vi "Main8.vi"() -> ()   [LabVIEW 2017]
uses:
  <vilib>/Analysis/2dsp.llb/Real FFT.vi
  <vilib>/Analysis/NI_AALPro.lvlib
  Atmcd32d.dll
panel:
  in  "index (row)":i32
  out "Angle Integrated Spectrum 2":T1(graph)
  in  "Area Parameteres":T2={"Center angle (deg)"=90.0, "Arc length (deg)"=90.0, "Angle step (deg)"=10.0, "Outer radius "=0.7640449438202247, "Inner radius "=0.0, "Radius"=0.0, "Radial step "=0.5}
  in  "Tab Control":T3(tab)
  out "Current angle":dbl
  in  "Exposure time [ms]":u32=100
  out "Count":i32
  in  "Integration time [s]":dbl=1.0
  out "Ready":bool
  out "Connected":bool
  out "Device":refnum<visa-resource-name>
  in  "Exit":bool
  in  "Take image":bool
  in  "Spectrum":T4(tab)
  out "Fully Integrated Spectrum":dbl(graph)
  out "Angular distribution":dbl[][](graph)
  out "Angle Integrated Spectrum":T5(graph)
  out "Angular distribution 2":dbl[][](graph)
  in  "Energy/Radius":enum32{"Radius", "Energy"}(radio)
  out "Spectrogram up":dbl[][](graph)=[[0.0010313840536425023, 0.0010313840536425023, 0.0010274759814052766, 0.0010401531177745159, 0.00104452387932524, 0.0010522711712232782, 0.001047206375702307, 0.0010453914217880493, 0.0010393489196820073, 0.0010272942106035452, 0.0010408196107141979, 0.0010468510964080136, 0.001062026204249532, 0.001106433361933133, 0.001154520001300267, 0.0011934960677563772, 0.001214033414248973, 0.0012241024150236718, 0.0012391453259184763, 0.0012555680424446059, 0.0012925281054633312, 0.001352528994653044, 0.0014089853532089937, 0.0014660421062312687, 0.0015363130457188075, 0.0015691474623588406, 0.0016108363203256395, 0.0016140062929437132, 0.0015863330654316305, 0.001566139981821102, 0.0015480455247396548, 0.0015630250912641588, 0.0016089194645982896, 0.0016388896140595243, 0.0016752961023638853, 0.001688323009821305, 0.0016919033437948032, 0.0017147706614732288, 0.0017464097973867246, 0.001779717919752482, 0.001837171263614898, 0.00188523587015758, 0.001909243386501412, 0.0019293676175355272, 0.0019505631946586353, 0.0019533283141273984, 0.001977616748982997, 0.0019911972311547808, 0.002017708227177005, 0.002053718124641225, 0.0020883013967221585, 0.002112669700566397, 0.0021315656016372966, 0.0021208218456137463, 0.002105299720787104, 0.002099830072116822, 0.0021012126318512036, 0.0020908214010188896, 0.002095054457416787, 0.002100080695494967, 0.0021084586769929523, 0.0020993728910094368, 0.002104955457905037, 0.0020792872174181134, 0.0020928346503532183, 0.0020942117018814864, 0.002102964241395161, 0.0021093372358679877, 0.002121036665652156, 0.002136567052787968, 0.002154127213876447, 0.002169360157882152, 0.0021869395976920275, 0.0021825908689657556, 0.002171045668952753, 0.0021674267775364637, 0.0021489908116760054, 0.002157660728097984, 0.002145658346977596, 0.002135917084466625, 0.00209696855904108, 0.0020850653256307278, 0.0020535996982097935, 0.002049595232365589, 0.0020524236962046524, 0.0020767176392663643, 0.002111884781195284, 0.002137809153266466, 0.0021668842192343256, 0.00216397037820051, 0.0021656008072099796, 0.0021352698702483386, 0.0021013916485498785, 0.0020823029602650214, 0.0020479290000163844, 0.0020333460243320213, 0.0020002169186649392, 0.0019659586307446764, 0.0019358700548520106, 0.0019274369912928948, 0.0019173046461478957, 0.001900014387158957, 0.0018599917615413628, 0.001814549061108504, 0.0017608991335671654, 0.0017321325271416374, 0.0017011240808280886, 0.0016809695546603515, 0.0016804848325224012, 0.001677022924980334, 0.0016912533754734602, 0.0016999535870290603, 0.0017145172839920274, 0.001701024933118053, 0.0017087557003977521, 0.0017038864461937952, 0.0017154509249281934, 0.0017378638156022909, 0.001773105318313737, 0.0017971238510697952, 0.001824766783448256, 0.0018273914436611356, 0.0018233456662710829, 0.001811169776658133, 0.001808649772361402, 0.0017980740166243004, 0.0017838545825434003, 0.001763256645783561, 0.0017210445082360198, 0.001701132343137258, 0.0016754062664861471, 0.001664623953019805, 0.0016487024832499652, 0.0016273141189128994, 0.0016010950578146683, 0.0015728930425157306, 0.0015352912734848325, 0.0015149109108664593, 0.001483448037548582, 0.0014523514599372237, 0.0014315579818603703, 0.0014274984339550348, 0.0014181675327994876, 0.0014143999198181453, 0.0014053113797315735, 0.0013993515007172275, 0.001408693418285001, 0.0013985390403155494, 0.001397974449188959, 0.0013917694550025816, 0.0013787315311329358, 0.0013626448151797038, 0.0013449083914956062, 0.0013370509354753064, 0.001325880293477993, 0.0013185543793476045, 0.001294420174263172, 0.00127875483607759, 0.0012659041912157889, 0.0012433398248735822, 0.001228894554342046, 0.0012003400138518715, 0.001183988904005212, 0.0011747543964566436, 0.0011585547622780935, 0.0011605046672421217, 0.0011473565792502146, 0.0011370039058606926, 0.0011340652778993677, 0.0011226770617605876, 0.0011216442731143861, 0.0011107600578349525, 0.0011026409620242816, 0.0010866919512238764, 0.0010731362559796018, 0.001051089661012024, 0.0010301832647098524, 0.001009888279286232, 0.0009965887156262153, 0.0009909235256389188, 0.0009767536654130364, 0.0009747817276245561, 0.0009568910741692924, 0.000949947980363763, 0.000956703795161448, 0.0009593917997446279, 0.0009746082191319944, 0.0009815127554947322, 0.0009862085012061277, 0.0009848589907084247, 0.0009587748806599638, 0.0009397330121270677, 0.0009244532483694009, 0.0009160174307072283, 0.0009138141482619988, 0.0009141501488348964, 0.0009184162544694721, 0.0009130457535092251, 0.000912208506180038, 0.0009004897976744733, 0.0008954966088329721, 0.000888658170943591, 0.000878327530378521, 0.0008779392018475493, 0.0008724833236925496, 0.0008753007711193868, 0.0008733894235981503, 0.0008842763929806406, 0.0008803270091975667, 0.0008834474079606231, 0.0008812331091031674, 0.0008784927765619131, 0.0008838109495640858, 0.0008909550928927427, 0.000899184352825675, 0.0009081654828930417, 0.000914194214483801, 0.0009259542345352136, 0.0009387635678511666, 0.0009425339349355657, 0.0009425063939050002, 0.0009326494590656548, 0.0009267529244216092, 0.0009192645182108854, 0.0009126023429171226, 0.0009054058716303917, 0.0008956756255316468, 0.0008975015958581308, 0.0008902445343041561, 0.0008840973762819658, 0.0008824283898297043, 0.0008799772381093866, 0.000884678492026895, 0.0008933897199947213, 0.0008983829088362226, 0.000893860671617389, 0.0008973749071175302, 0.0009013435696219998, 0.0009055848883290665, 0.0009138995254567515, 0.0009202174378684471, 0.000930589389979365, 0.000922150818214136, 0.0009280666315795773, 0.0009267253833910438, 0.0009243623629685353, 0.0009317653919845064, 0.0009418922289233926, 0.0009494384712983037, 0.0009643051195974898, 0.0009718458537662879, 0.0009862966325039368, 0.0009917001827008621, 0.0009979795376697665, 0.001014038712592433, 0.0010172830459930335, 0.0010330585483008768, 0.0010469640146333317, 0.001060098332109956, 0.0010826544361429932, 0.0011030761103072145, 0.0011350760337211167, 0.0011531154087414334, 0.0011576624328877758, 0.0011768364983673857, 0.0011841624124977737, 0.0011999406689086737, 0.0012165093528967996, 0.0012281895039595726, 0.0012561601746017613, 0.0012707651831105765, 0.001307240523991351, 0.001333627585376031, 0.0013666217399933432, 0.0014024911782016796, 0.0014332324765187446, 0.0014678102403935655, 0.0014988241949132272, 0.0015329365153714935, 0.0015343879276822883, 0.0015720971067323913, 0.0016118636007657278, 0.001651087536496926, 0.0016970920739533186, 0.001745473402347502, 0.0017665615694514051, 0.0018051024876245825, 0.0018256783915599696, 0.0018815618966801597, 0.0018972630382054765, 0.0019475088943689358, 0.001967589059754146, 0.0019944801219981727, 0.0020293085092511383, 0.0020797967264835726, 0.002127649267090901, 0.002177592171918141, 0.002209096356781867, 0.0022576126362258207, 0.0022860239633570555, 0.002367479315357191, 0.00239798651491445, 0.002459918030346795, 0.002492961758819125, 0.0025305745442622493, 0.0025619850896220525, 0.0025918974029190997, 0.0026126908809959533, 0.0026649499864937407, 0.002671884817990101, 0.0027487573425041584, 0.0027664331759210126, 0.0028080311484869457, 0.002835572179052315, 0.002897776350687257, 0.0029281981730497637, 0.0029626547563900967, 0.002993387792397992, 0.0030170785868903222, 0.0030149964849795806, 0.0030319039236436605, 0.0030360240618162396, 0.0030334957952103388, 0.0030378693108641195, 0.003026379192912247, 0.0030242502712495446, 0.0030348563221202682, 0.0030418489897808152, 0.0030719182869520852, 0.0030982750532031434, 0.0030908086798168716, 0.0031010319103627363, 0.0031036813575031253, 0.0030762670156783568, 0.003066933360419753, 0.003042223547796504, 0.0030263378813663996, 0.003004663090311454, 0.0029920548065186284, 0.0029706664421815625, 0.0029578268137319874, 0.0029413352446294445, 0.0029132489016588815, 0.0028961762168114094, 0.002857943758180564, 0.00283680050901553, 0.0028030104186148787, 0.0027938640423641197, 0.0027516161014768444, 0.002719478472910115, 0.0026733913123620267, 0.002627637398283779, 0.0025728335015617514, 0.0025436510255746865, 0.002504355483164018, 0.0024615594757684913, 0.002436053727361903, 0.0024182842544411267, 0.0024007185851465346, 0.0023905779776923655, 0.0023550968680150007, 0.002333292634116398, 0.002292746728918062, 0.0022553735504408563, 0.0022384468330553806, 0.002203128215458351, 0.00217902430550754, 0.002143711196116624, 0.0021122262899742946, 0.0020506142504965077, 0.00203825383597877, 0.0020262487007553258, 0.0020074629638066875, 0.0019932738248594093, 0.0019544327094530695, 0.0019488088310116213, 0.0019049882972790627, 0.0018915620448784454, 0.0018528393559035367, 0.001821197465886984, 0.0017890212798774634, 0.0017354539754278208, 0.0016897689139259869, 0.001663423164087155, 0.0016456371665480398, 0.0016412085688331283, 0.001628644350689207, 0.0016130809143167168, 0.0016073331012377244, 0.001603339651805746, 0.0015941712427305346, 0.001588935692820058, 0.0015824029603699523, 0.00157714813173808, 0.0015643332902160138, 0.0015630746651191763, 0.0015527274999357675, 0.0015555421932595482, 0.0015637163711313498, 0.0015732180266764021, 0.001592557338339404, 0.001584653062567143, 0.0015960522951181493, 0.0016165015103129358, 0.0016268707083207973, 0.0016398039762742945, 0.001641899848700319, 0.0016484215647381982, 0.0016487190078683044, 0.0016555629539637985, 0.0016557612493838694, 0.0016741145921526312, 0.0017004658501975761, 0.0017330110860166727, 0.0017605190673453631, 0.0017664348807108045, 0.0017779084740443371, 0.001790398331405732, 0.0018131775177863488, 0.0018366452299310996, 0.0018605453362557267, 0.0018882543671075445, 0.0018984252696953353, 0.001914192509694009, 0.0019416316384462862, 0.0019781785860065308, 0.0020108477564631713, 0.0020298097560074277, 0.0020661143424986973, 0.002068810609391047, 0.002110609631480107, 0.002115869968318093, 0.0021256800834054774, 0.0021556667574850513, 0.002178443189762611, 0.0021840174943490416, 0.002213334921385877, 0.002212183706308245, 0.00223874152208243, 0.0022391546375409104, 0.002258397555596934, 0.0022739802706908193, 0.0023094503639559585, 0.002319709397841558, 0.002351866305129683, 0.002368812301236555, 0.0023749456887434623, 0.002389630566240917, 0.0023986777947816403, 0.00241149814450982, 0.0024190003212358263, 0.0024229882624616918, 0.002422095933071374, 0.002423731870286957, 0.0024201625527256847, 0.0024417767535133868, 0.0024415812121963724, 0.002455808908586442, 0.002457513698378438, 0.0024465385976981386, 0.0024522313287160006, 0.0024169705472831585, 0.0024148361174143426, 0.0023995701241719585, 0.0023793853028705996, 0.0023548297200185167, 0.002332361747283289, 0.0023205108418310103, 0.0022940521737668603, 0.0022523164960481005, 0.0022274744864781374, 0.0022039158889325208, 0.0021684926154193433, 0.0021411526343771015, 0.002118635087786856, 0.002083801192327777, 0.002047124801923875, 0.0020278653592495127, 0.0019697703093749233, 0.0019519264756716211, 0.0019212622922401392, 0.0018812286502103187, 0.0018427428140982722, 0.001812265909674635, 0.00175640994558501, 0.0017214080498394828, 0.0016736711815605288, 0.0016349457384825634, 0.0015946835058990505, 0.0015675610989982752, 0.0015259052902681545, 0.0014996366553149056, 0.001476708747369236, 0.001439175830914751, 0.0014011692087345419, 0.0013630882257718063, 0.0013162216540587178, 0.0012905451512626243, 0.0012539458757443056, 0.0012235736272368167, 0.0012001196856073486, 0.001185272316029558, 0.0011544346241055146, 0.0011379100057662933, 0.0010844501113358553, 0.0010647610285846733, 0.0010130802847287583, 0.0009929670701068693, 0.0009656849252288149, 0.0009476042386626501, 0.0009280005331062204, 0.0009123489654359212, 0.0008921173243826012, 0.0008740696870531149, 0.000861342976828858, 0.0008399518583887359, 0.0008269304591374295, 0.000805963472568014, 0.0007840931401960546, 0.0007730684656607372, 0.0007618757908389714, 0.000755502796366145, 0.0007484440302322409, 0.0007361304354664644, 0.0007236515945172958, 0.0007035631668229157, 0.0006909796699575985, 0.0006775396470416985, 0.0006603843391025302, 0.0006506954045496334, 0.0006404831904159946, 0.0006315406177914192, 0.000626814576946402, 0.0006201799426832045, 0.0006156053775062967, 0.0006078663479174281, 0.0005998298751984535, 0.0005900335306263518, 0.0005812644664943382, 0.0005748804556092857, 0.0005698349388097101, 0.000566761359798615, 0.0005616442363195694, 0.0005622749259195163, 0.0005532993040582626, 0.0005422911541412846, 0.0005348495676825219, 0.0005325361211150309, 0.0005320376284617976, 0.0005307018884793774, 0.0005264054877111798, 0.0005264054877111798, 0.0005228637111804734, 0.0005181238998201733, 0.0005176309153730532, 0.0005136154331166225, 0.0005124091359778592, 0.0005101562796776121, 0.0005055431570579128, 0.0004995529829099451, 0.0004920150028442035, 0.0004884759804165536, 0.00048560345092858563, 0.000481450263519328, 0.000479029406932632, 0.00047415189041950524, 0.00047243608421528277, 0.0004715299843096821, 0.00047353772543789753, 0.00047000971942247376, 0.0004698554896513077, 0.0004721276246729506, 0.0004682388311571205, 0.0004696351614067847, 0.0004644106279085342, 0.00046173088563452376, 0.0004594807834373332, 0.0004550053659704607, 0.0004509155229315034, 0.00044808430498938354, 0.0004430277717775818, 0.0004410696045043841, 0.00043787759906185783, 0.00043347929648056836, 0.0004299017166101269, 0.00042542354504019795, 0.00042215993291820175, 0.00041868425486085215, 0.000416883071461877, 0.0004110388647759057, 0.0004118981449295452, 0.00040788541677617095, 0.00040867033614728403, 0.00040761000647051725, 0.0004041866563712419, 0.00040178507850594175, 0.00039903372955246133, 0.0003977007436730975, 0.0003977310388067194, 0.00039884645054461687, 0.00039690480788975835, 0.000394671230310907, 0.0003933712936682215, 0.00039117076532604856, 0.0003899947633209073, 0.00038895095826247983, 0.00038990112381698505, 0.00038822662915861066, 0.0003852577060636639, 0.00038354740806555447, 0.0003831673418437523, 0.00038108523993301045, 0.00038199133983861106, 0.0003807712721845652, 0.0003789921216100424, 0.0003772350038599718, 0.00037759028315426514, 0.0003756155912627282, 0.0003736216206497954, 0.000373136898511845, 0.0003710079768491419, 0.0003707132878220925, 0.0003699917128212798, 0.00036924259678990177, 0.0003697686304737003, 0.000369484957858877, 0.0003692976788510325, 0.00037006056539769325, 0.00036974108944313496, 0.00036845492331573224, 0.0003671825277036122, 0.0003674441674939832, 0.00036729820003198675, 0.00036671708428705744, 0.0003670723635813507, 0.0003662516408705027, 0.0003653593114801848, 0.0003654336722627113, 0.00036621859163382426, 0.0003649076385789127, 0.0003645000313265452, 0.00036404009611610357, 0.00036481399907499045, 0.00036354435756592694, 0.0003624454704463687, 0.00036318632416857717, 0.000362616224835874, 0.00036201858447260554, 0.0003629026515537539, 0.00036316429134412485, 0.0003618092726403087, 0.00036178173160974337, 0.0003609059268377646, 0.0003606580575626763, 0.00035972441662651027, 0.00035978776099681063, 0.0003598290725426587, 0.0003593278257863689, 0.00035902487445014993, 0.0003587962838964574, 0.00035836939792269413, 0.00035583837721373673, 0.0003554059830338604, 0.0003547532606094612, 0.0003549102444836838, 0.00035429057129596295, 0.0003543126041204152, 0.0003549185067928534, 0.0003548248672889311, 0.00035513057272820676, 0.0003544998831282598, 0.00035434014515098067, 0.000354516407746599, 0.00035333489753534467, 0.0003535855209134895, 0.0003530154215807864, 0.0003527152243476239, 0.0003532798154742139, 0.00035263260125592777, 0.0003519964034498677, 0.000351608074918896, 0.00035093882787615757, 0.000349443349916458, 0.00034942957940117537, 0.0003491624314046913, 0.00034956453045094566, 0.00034901095573658175, 0.00034910184113744744, 0.0003489310867479422, 0.0003488181685226241, 0.0003479836752964935, 0.0003476917403725006, 0.00034843259409470895, 0.0003489586277785075, 0.0003480910853156984, 0.0003474548875096384, 0.0003469619030625183, 0.00034665344352018617, 0.0003463918037298151, 0.00034654052529486815, 0.00034605304905386115, 0.0003454196053508576, 0.00034516347376659963, 0.00034559862204953256, 0.0003448357355028718, 0.0003449403914190202, 0.00034430419361296017, 0.00034424635744877293, 0.000344852260121211, 0.0003448384896059283, 0.0003451028834993559, 0.0003437423565894266, 0.0003425580922751158, 0.00034259664971790727, 0.0003416354677511759, 0.00034174838597649394, 0.00034173461546121124, 0.0003417869434192854, 0.0003409965158420593, 0.00034094143378092864, 0.0003408477942770064, 0.0003402501539137379, 0.0003404980231888262, 0.0003398783500011054, 0.00033904936498108774, 0.00033842969179336696, 0.00033828372433137053, 0.0003380661501899041, 0.00033740791955939176, 0.000338358085113897, 0.0003377081167925543, 0.00033727847671573453, 0.000337388640837996, 0.00033701959102842003, 0.00033749605085720095, 0.00033774116602923275, 0.0003364384752834908, 0.000335931720321088, 0.0003357031297673954, 0.00033592070390886183, 0.0003353395881639325, 0.00033492922680850853, 0.00033513303043469225, 0.00033468961984258985, 0.0003348713906443213, 0.00033494024322073466, 0.0003348108003770775, 0.00033487689885043436, 0.00033441145543387964, 0.0003341993894985263, 0.0003345464064836499, 0.00033424896335354395, 0.00033390194636842026, 0.00033334837165405635, 0.00033337040447850867, 0.0003331583385431553, 0.0003329132233711235, 0.0003332326993256818, 0.0003335301424557878, 0.0003335026014252224, 0.00033401761869679484, 0.0003333428634479433, 0.00033282509207331433, 0.00033313630571870306, 0.0003330839777606288, 0.00033270666564188324, 0.00033214758272140626, 0.00033204843501137094, 0.00033124974512497527, 0.0003311781384455053, 0.00033189695934326144, 0.0003313213518044452, 0.0003320980088663886, 0.0003318336149729611, 0.00033207873014499283, 0.0003325304030462649, 0.0003314094831022544, 0.00033175650008737803]]
  out "Range scan":dbl[][](graph)
  out "Spectrogram down":dbl[][](graph)=[[0.0010313840536425023, 0.0010313840536425023, 0.0010274759814052766, 0.0010401531177745159, 0.00104452387932524, 0.0010522711712232782, 0.001047206375702307, 0.0010453914217880493, 0.0010393489196820073, 0.0010272942106035452, 0.0010408196107141979, 0.0010468510964080136, 0.001062026204249532, 0.001106433361933133, 0.001154520001300267, 0.0011934960677563772, 0.001214033414248973, 0.0012241024150236718, 0.0012391453259184763, 0.0012555680424446059, 0.0012925281054633312, 0.001352528994653044, 0.0014089853532089937, 0.0014660421062312687, 0.0015363130457188075, 0.0015691474623588406, 0.0016108363203256395, 0.0016140062929437132, 0.0015863330654316305, 0.001566139981821102, 0.0015480455247396548, 0.0015630250912641588, 0.0016089194645982896, 0.0016388896140595243, 0.0016752961023638853, 0.001688323009821305, 0.0016919033437948032, 0.0017147706614732288, 0.0017464097973867246, 0.001779717919752482, 0.001837171263614898, 0.00188523587015758, 0.001909243386501412, 0.0019293676175355272, 0.0019505631946586353, 0.0019533283141273984, 0.001977616748982997, 0.0019911972311547808, 0.002017708227177005, 0.002053718124641225, 0.0020883013967221585, 0.002112669700566397, 0.0021315656016372966, 0.0021208218456137463, 0.002105299720787104, 0.002099830072116822, 0.0021012126318512036, 0.0020908214010188896, 0.002095054457416787, 0.002100080695494967, 0.0021084586769929523, 0.0020993728910094368, 0.002104955457905037, 0.0020792872174181134, 0.0020928346503532183, 0.0020942117018814864, 0.002102964241395161, 0.0021093372358679877, 0.002121036665652156, 0.002136567052787968, 0.002154127213876447, 0.002169360157882152, 0.0021869395976920275, 0.0021825908689657556, 0.002171045668952753, 0.0021674267775364637, 0.0021489908116760054, 0.002157660728097984, 0.002145658346977596, 0.002135917084466625, 0.00209696855904108, 0.0020850653256307278, 0.0020535996982097935, 0.002049595232365589, 0.0020524236962046524, 0.0020767176392663643, 0.002111884781195284, 0.002137809153266466, 0.0021668842192343256, 0.00216397037820051, 0.0021656008072099796, 0.0021352698702483386, 0.0021013916485498785, 0.0020823029602650214, 0.0020479290000163844, 0.0020333460243320213, 0.0020002169186649392, 0.0019659586307446764, 0.0019358700548520106, 0.0019274369912928948, 0.0019173046461478957, 0.001900014387158957, 0.0018599917615413628, 0.001814549061108504, 0.0017608991335671654, 0.0017321325271416374, 0.0017011240808280886, 0.0016809695546603515, 0.0016804848325224012, 0.001677022924980334, 0.0016912533754734602, 0.0016999535870290603, 0.0017145172839920274, 0.001701024933118053, 0.0017087557003977521, 0.0017038864461937952, 0.0017154509249281934, 0.0017378638156022909, 0.001773105318313737, 0.0017971238510697952, 0.001824766783448256, 0.0018273914436611356, 0.0018233456662710829, 0.001811169776658133, 0.001808649772361402, 0.0017980740166243004, 0.0017838545825434003, 0.001763256645783561, 0.0017210445082360198, 0.001701132343137258, 0.0016754062664861471, 0.001664623953019805, 0.0016487024832499652, 0.0016273141189128994, 0.0016010950578146683, 0.0015728930425157306, 0.0015352912734848325, 0.0015149109108664593, 0.001483448037548582, 0.0014523514599372237, 0.0014315579818603703, 0.0014274984339550348, 0.0014181675327994876, 0.0014143999198181453, 0.0014053113797315735, 0.0013993515007172275, 0.001408693418285001, 0.0013985390403155494, 0.001397974449188959, 0.0013917694550025816, 0.0013787315311329358, 0.0013626448151797038, 0.0013449083914956062, 0.0013370509354753064, 0.001325880293477993, 0.0013185543793476045, 0.001294420174263172, 0.00127875483607759, 0.0012659041912157889, 0.0012433398248735822, 0.001228894554342046, 0.0012003400138518715, 0.001183988904005212, 0.0011747543964566436, 0.0011585547622780935, 0.0011605046672421217, 0.0011473565792502146, 0.0011370039058606926, 0.0011340652778993677, 0.0011226770617605876, 0.0011216442731143861, 0.0011107600578349525, 0.0011026409620242816, 0.0010866919512238764, 0.0010731362559796018, 0.001051089661012024, 0.0010301832647098524, 0.001009888279286232, 0.0009965887156262153, 0.0009909235256389188, 0.0009767536654130364, 0.0009747817276245561, 0.0009568910741692924, 0.000949947980363763, 0.000956703795161448, 0.0009593917997446279, 0.0009746082191319944, 0.0009815127554947322, 0.0009862085012061277, 0.0009848589907084247, 0.0009587748806599638, 0.0009397330121270677, 0.0009244532483694009, 0.0009160174307072283, 0.0009138141482619988, 0.0009141501488348964, 0.0009184162544694721, 0.0009130457535092251, 0.000912208506180038, 0.0009004897976744733, 0.0008954966088329721, 0.000888658170943591, 0.000878327530378521, 0.0008779392018475493, 0.0008724833236925496, 0.0008753007711193868, 0.0008733894235981503, 0.0008842763929806406, 0.0008803270091975667, 0.0008834474079606231, 0.0008812331091031674, 0.0008784927765619131, 0.0008838109495640858, 0.0008909550928927427, 0.000899184352825675, 0.0009081654828930417, 0.000914194214483801, 0.0009259542345352136, 0.0009387635678511666, 0.0009425339349355657, 0.0009425063939050002, 0.0009326494590656548, 0.0009267529244216092, 0.0009192645182108854, 0.0009126023429171226, 0.0009054058716303917, 0.0008956756255316468, 0.0008975015958581308, 0.0008902445343041561, 0.0008840973762819658, 0.0008824283898297043, 0.0008799772381093866, 0.000884678492026895, 0.0008933897199947213, 0.0008983829088362226, 0.000893860671617389, 0.0008973749071175302, 0.0009013435696219998, 0.0009055848883290665, 0.0009138995254567515, 0.0009202174378684471, 0.000930589389979365, 0.000922150818214136, 0.0009280666315795773, 0.0009267253833910438, 0.0009243623629685353, 0.0009317653919845064, 0.0009418922289233926, 0.0009494384712983037, 0.0009643051195974898, 0.0009718458537662879, 0.0009862966325039368, 0.0009917001827008621, 0.0009979795376697665, 0.001014038712592433, 0.0010172830459930335, 0.0010330585483008768, 0.0010469640146333317, 0.001060098332109956, 0.0010826544361429932, 0.0011030761103072145, 0.0011350760337211167, 0.0011531154087414334, 0.0011576624328877758, 0.0011768364983673857, 0.0011841624124977737, 0.0011999406689086737, 0.0012165093528967996, 0.0012281895039595726, 0.0012561601746017613, 0.0012707651831105765, 0.001307240523991351, 0.001333627585376031, 0.0013666217399933432, 0.0014024911782016796, 0.0014332324765187446, 0.0014678102403935655, 0.0014988241949132272, 0.0015329365153714935, 0.0015343879276822883, 0.0015720971067323913, 0.0016118636007657278, 0.001651087536496926, 0.0016970920739533186, 0.001745473402347502, 0.0017665615694514051, 0.0018051024876245825, 0.0018256783915599696, 0.0018815618966801597, 0.0018972630382054765, 0.0019475088943689358, 0.001967589059754146, 0.0019944801219981727, 0.0020293085092511383, 0.0020797967264835726, 0.002127649267090901, 0.002177592171918141, 0.002209096356781867, 0.0022576126362258207, 0.0022860239633570555, 0.002367479315357191, 0.00239798651491445, 0.002459918030346795, 0.002492961758819125, 0.0025305745442622493, 0.0025619850896220525, 0.0025918974029190997, 0.0026126908809959533, 0.0026649499864937407, 0.002671884817990101, 0.0027487573425041584, 0.0027664331759210126, 0.0028080311484869457, 0.002835572179052315, 0.002897776350687257, 0.0029281981730497637, 0.0029626547563900967, 0.002993387792397992, 0.0030170785868903222, 0.0030149964849795806, 0.0030319039236436605, 0.0030360240618162396, 0.0030334957952103388, 0.0030378693108641195, 0.003026379192912247, 0.0030242502712495446, 0.0030348563221202682, 0.0030418489897808152, 0.0030719182869520852, 0.0030982750532031434, 0.0030908086798168716, 0.0031010319103627363, 0.0031036813575031253, 0.0030762670156783568, 0.003066933360419753, 0.003042223547796504, 0.0030263378813663996, 0.003004663090311454, 0.0029920548065186284, 0.0029706664421815625, 0.0029578268137319874, 0.0029413352446294445, 0.0029132489016588815, 0.0028961762168114094, 0.002857943758180564, 0.00283680050901553, 0.0028030104186148787, 0.0027938640423641197, 0.0027516161014768444, 0.002719478472910115, 0.0026733913123620267, 0.002627637398283779, 0.0025728335015617514, 0.0025436510255746865, 0.002504355483164018, 0.0024615594757684913, 0.002436053727361903, 0.0024182842544411267, 0.0024007185851465346, 0.0023905779776923655, 0.0023550968680150007, 0.002333292634116398, 0.002292746728918062, 0.0022553735504408563, 0.0022384468330553806, 0.002203128215458351, 0.00217902430550754, 0.002143711196116624, 0.0021122262899742946, 0.0020506142504965077, 0.00203825383597877, 0.0020262487007553258, 0.0020074629638066875, 0.0019932738248594093, 0.0019544327094530695, 0.0019488088310116213, 0.0019049882972790627, 0.0018915620448784454, 0.0018528393559035367, 0.001821197465886984, 0.0017890212798774634, 0.0017354539754278208, 0.0016897689139259869, 0.001663423164087155, 0.0016456371665480398, 0.0016412085688331283, 0.001628644350689207, 0.0016130809143167168, 0.0016073331012377244, 0.001603339651805746, 0.0015941712427305346, 0.001588935692820058, 0.0015824029603699523, 0.00157714813173808, 0.0015643332902160138, 0.0015630746651191763, 0.0015527274999357675, 0.0015555421932595482, 0.0015637163711313498, 0.0015732180266764021, 0.001592557338339404, 0.001584653062567143, 0.0015960522951181493, 0.0016165015103129358, 0.0016268707083207973, 0.0016398039762742945, 0.001641899848700319, 0.0016484215647381982, 0.0016487190078683044, 0.0016555629539637985, 0.0016557612493838694, 0.0016741145921526312, 0.0017004658501975761, 0.0017330110860166727, 0.0017605190673453631, 0.0017664348807108045, 0.0017779084740443371, 0.001790398331405732, 0.0018131775177863488, 0.0018366452299310996, 0.0018605453362557267, 0.0018882543671075445, 0.0018984252696953353, 0.001914192509694009, 0.0019416316384462862, 0.0019781785860065308, 0.0020108477564631713, 0.0020298097560074277, 0.0020661143424986973, 0.002068810609391047, 0.002110609631480107, 0.002115869968318093, 0.0021256800834054774, 0.0021556667574850513, 0.002178443189762611, 0.0021840174943490416, 0.002213334921385877, 0.002212183706308245, 0.00223874152208243, 0.0022391546375409104, 0.002258397555596934, 0.0022739802706908193, 0.0023094503639559585, 0.002319709397841558, 0.002351866305129683, 0.002368812301236555, 0.0023749456887434623, 0.002389630566240917, 0.0023986777947816403, 0.00241149814450982, 0.0024190003212358263, 0.0024229882624616918, 0.002422095933071374, 0.002423731870286957, 0.0024201625527256847, 0.0024417767535133868, 0.0024415812121963724, 0.002455808908586442, 0.002457513698378438, 0.0024465385976981386, 0.0024522313287160006, 0.0024169705472831585, 0.0024148361174143426, 0.0023995701241719585, 0.0023793853028705996, 0.0023548297200185167, 0.002332361747283289, 0.0023205108418310103, 0.0022940521737668603, 0.0022523164960481005, 0.0022274744864781374, 0.0022039158889325208, 0.0021684926154193433, 0.0021411526343771015, 0.002118635087786856, 0.002083801192327777, 0.002047124801923875, 0.0020278653592495127, 0.0019697703093749233, 0.0019519264756716211, 0.0019212622922401392, 0.0018812286502103187, 0.0018427428140982722, 0.001812265909674635, 0.00175640994558501, 0.0017214080498394828, 0.0016736711815605288, 0.0016349457384825634, 0.0015946835058990505, 0.0015675610989982752, 0.0015259052902681545, 0.0014996366553149056, 0.001476708747369236, 0.001439175830914751, 0.0014011692087345419, 0.0013630882257718063, 0.0013162216540587178, 0.0012905451512626243, 0.0012539458757443056, 0.0012235736272368167, 0.0012001196856073486, 0.001185272316029558, 0.0011544346241055146, 0.0011379100057662933, 0.0010844501113358553, 0.0010647610285846733, 0.0010130802847287583, 0.0009929670701068693, 0.0009656849252288149, 0.0009476042386626501, 0.0009280005331062204, 0.0009123489654359212, 0.0008921173243826012, 0.0008740696870531149, 0.000861342976828858, 0.0008399518583887359, 0.0008269304591374295, 0.000805963472568014, 0.0007840931401960546, 0.0007730684656607372, 0.0007618757908389714, 0.000755502796366145, 0.0007484440302322409, 0.0007361304354664644, 0.0007236515945172958, 0.0007035631668229157, 0.0006909796699575985, 0.0006775396470416985, 0.0006603843391025302, 0.0006506954045496334, 0.0006404831904159946, 0.0006315406177914192, 0.000626814576946402, 0.0006201799426832045, 0.0006156053775062967, 0.0006078663479174281, 0.0005998298751984535, 0.0005900335306263518, 0.0005812644664943382, 0.0005748804556092857, 0.0005698349388097101, 0.000566761359798615, 0.0005616442363195694, 0.0005622749259195163, 0.0005532993040582626, 0.0005422911541412846, 0.0005348495676825219, 0.0005325361211150309, 0.0005320376284617976, 0.0005307018884793774, 0.0005264054877111798, 0.0005264054877111798, 0.0005228637111804734, 0.0005181238998201733, 0.0005176309153730532, 0.0005136154331166225, 0.0005124091359778592, 0.0005101562796776121, 0.0005055431570579128, 0.0004995529829099451, 0.0004920150028442035, 0.0004884759804165536, 0.00048560345092858563, 0.000481450263519328, 0.000479029406932632, 0.00047415189041950524, 0.00047243608421528277, 0.0004715299843096821, 0.00047353772543789753, 0.00047000971942247376, 0.0004698554896513077, 0.0004721276246729506, 0.0004682388311571205, 0.0004696351614067847, 0.0004644106279085342, 0.00046173088563452376, 0.0004594807834373332, 0.0004550053659704607, 0.0004509155229315034, 0.00044808430498938354, 0.0004430277717775818, 0.0004410696045043841, 0.00043787759906185783, 0.00043347929648056836, 0.0004299017166101269, 0.00042542354504019795, 0.00042215993291820175, 0.00041868425486085215, 0.000416883071461877, 0.0004110388647759057, 0.0004118981449295452, 0.00040788541677617095, 0.00040867033614728403, 0.00040761000647051725, 0.0004041866563712419, 0.00040178507850594175, 0.00039903372955246133, 0.0003977007436730975, 0.0003977310388067194, 0.00039884645054461687, 0.00039690480788975835, 0.000394671230310907, 0.0003933712936682215, 0.00039117076532604856, 0.0003899947633209073, 0.00038895095826247983, 0.00038990112381698505, 0.00038822662915861066, 0.0003852577060636639, 0.00038354740806555447, 0.0003831673418437523, 0.00038108523993301045, 0.00038199133983861106, 0.0003807712721845652, 0.0003789921216100424, 0.0003772350038599718, 0.00037759028315426514, 0.0003756155912627282, 0.0003736216206497954, 0.000373136898511845, 0.0003710079768491419, 0.0003707132878220925, 0.0003699917128212798, 0.00036924259678990177, 0.0003697686304737003, 0.000369484957858877, 0.0003692976788510325, 0.00037006056539769325, 0.00036974108944313496, 0.00036845492331573224, 0.0003671825277036122, 0.0003674441674939832, 0.00036729820003198675, 0.00036671708428705744, 0.0003670723635813507, 0.0003662516408705027, 0.0003653593114801848, 0.0003654336722627113, 0.00036621859163382426, 0.0003649076385789127, 0.0003645000313265452, 0.00036404009611610357, 0.00036481399907499045, 0.00036354435756592694, 0.0003624454704463687, 0.00036318632416857717, 0.000362616224835874, 0.00036201858447260554, 0.0003629026515537539, 0.00036316429134412485, 0.0003618092726403087, 0.00036178173160974337, 0.0003609059268377646, 0.0003606580575626763, 0.00035972441662651027, 0.00035978776099681063, 0.0003598290725426587, 0.0003593278257863689, 0.00035902487445014993, 0.0003587962838964574, 0.00035836939792269413, 0.00035583837721373673, 0.0003554059830338604, 0.0003547532606094612, 0.0003549102444836838, 0.00035429057129596295, 0.0003543126041204152, 0.0003549185067928534, 0.0003548248672889311, 0.00035513057272820676, 0.0003544998831282598, 0.00035434014515098067, 0.000354516407746599, 0.00035333489753534467, 0.0003535855209134895, 0.0003530154215807864, 0.0003527152243476239, 0.0003532798154742139, 0.00035263260125592777, 0.0003519964034498677, 0.000351608074918896, 0.00035093882787615757, 0.000349443349916458, 0.00034942957940117537, 0.0003491624314046913, 0.00034956453045094566, 0.00034901095573658175, 0.00034910184113744744, 0.0003489310867479422, 0.0003488181685226241, 0.0003479836752964935, 0.0003476917403725006, 0.00034843259409470895, 0.0003489586277785075, 0.0003480910853156984, 0.0003474548875096384, 0.0003469619030625183, 0.00034665344352018617, 0.0003463918037298151, 0.00034654052529486815, 0.00034605304905386115, 0.0003454196053508576, 0.00034516347376659963, 0.00034559862204953256, 0.0003448357355028718, 0.0003449403914190202, 0.00034430419361296017, 0.00034424635744877293, 0.000344852260121211, 0.0003448384896059283, 0.0003451028834993559, 0.0003437423565894266, 0.0003425580922751158, 0.00034259664971790727, 0.0003416354677511759, 0.00034174838597649394, 0.00034173461546121124, 0.0003417869434192854, 0.0003409965158420593, 0.00034094143378092864, 0.0003408477942770064, 0.0003402501539137379, 0.0003404980231888262, 0.0003398783500011054, 0.00033904936498108774, 0.00033842969179336696, 0.00033828372433137053, 0.0003380661501899041, 0.00033740791955939176, 0.000338358085113897, 0.0003377081167925543, 0.00033727847671573453, 0.000337388640837996, 0.00033701959102842003, 0.00033749605085720095, 0.00033774116602923275, 0.0003364384752834908, 0.000335931720321088, 0.0003357031297673954, 0.00033592070390886183, 0.0003353395881639325, 0.00033492922680850853, 0.00033513303043469225, 0.00033468961984258985, 0.0003348713906443213, 0.00033494024322073466, 0.0003348108003770775, 0.00033487689885043436, 0.00033441145543387964, 0.0003341993894985263, 0.0003345464064836499, 0.00033424896335354395, 0.00033390194636842026, 0.00033334837165405635, 0.00033337040447850867, 0.0003331583385431553, 0.0003329132233711235, 0.0003332326993256818, 0.0003335301424557878, 0.0003335026014252224, 0.00033401761869679484, 0.0003333428634479433, 0.00033282509207331433, 0.00033313630571870306, 0.0003330839777606288, 0.00033270666564188324, 0.00033214758272140626, 0.00033204843501137094, 0.00033124974512497527, 0.0003311781384455053, 0.00033189695934326144, 0.0003313213518044452, 0.0003320980088663886, 0.0003318336149729611, 0.00033207873014499283, 0.0003325304030462649, 0.0003314094831022544, 0.00033175650008737803]]
  out "FFT":dbl[](graph)
  out "Asymetry spectrogarm":dbl[][](graph)=[[0.0010313840536425023, 0.0010313840536425023, 0.0010274759814052766, 0.0010401531177745159, 0.00104452387932524, 0.0010522711712232782, 0.001047206375702307, 0.0010453914217880493, 0.0010393489196820073, 0.0010272942106035452, 0.0010408196107141979, 0.0010468510964080136, 0.001062026204249532, 0.001106433361933133, 0.001154520001300267, 0.0011934960677563772, 0.001214033414248973, 0.0012241024150236718, 0.0012391453259184763, 0.0012555680424446059, 0.0012925281054633312, 0.001352528994653044, 0.0014089853532089937, 0.0014660421062312687, 0.0015363130457188075, 0.0015691474623588406, 0.0016108363203256395, 0.0016140062929437132, 0.0015863330654316305, 0.001566139981821102, 0.0015480455247396548, 0.0015630250912641588, 0.0016089194645982896, 0.0016388896140595243, 0.0016752961023638853, 0.001688323009821305, 0.0016919033437948032, 0.0017147706614732288, 0.0017464097973867246, 0.001779717919752482, 0.001837171263614898, 0.00188523587015758, 0.001909243386501412, 0.0019293676175355272, 0.0019505631946586353, 0.0019533283141273984, 0.001977616748982997, 0.0019911972311547808, 0.002017708227177005, 0.002053718124641225, 0.0020883013967221585, 0.002112669700566397, 0.0021315656016372966, 0.0021208218456137463, 0.002105299720787104, 0.002099830072116822, 0.0021012126318512036, 0.0020908214010188896, 0.002095054457416787, 0.002100080695494967, 0.0021084586769929523, 0.0020993728910094368, 0.002104955457905037, 0.0020792872174181134, 0.0020928346503532183, 0.0020942117018814864, 0.002102964241395161, 0.0021093372358679877, 0.002121036665652156, 0.002136567052787968, 0.002154127213876447, 0.002169360157882152, 0.0021869395976920275, 0.0021825908689657556, 0.002171045668952753, 0.0021674267775364637, 0.0021489908116760054, 0.002157660728097984, 0.002145658346977596, 0.002135917084466625, 0.00209696855904108, 0.0020850653256307278, 0.0020535996982097935, 0.002049595232365589, 0.0020524236962046524, 0.0020767176392663643, 0.002111884781195284, 0.002137809153266466, 0.0021668842192343256, 0.00216397037820051, 0.0021656008072099796, 0.0021352698702483386, 0.0021013916485498785, 0.0020823029602650214, 0.0020479290000163844, 0.0020333460243320213, 0.0020002169186649392, 0.0019659586307446764, 0.0019358700548520106, 0.0019274369912928948, 0.0019173046461478957, 0.001900014387158957, 0.0018599917615413628, 0.001814549061108504, 0.0017608991335671654, 0.0017321325271416374, 0.0017011240808280886, 0.0016809695546603515, 0.0016804848325224012, 0.001677022924980334, 0.0016912533754734602, 0.0016999535870290603, 0.0017145172839920274, 0.001701024933118053, 0.0017087557003977521, 0.0017038864461937952, 0.0017154509249281934, 0.0017378638156022909, 0.001773105318313737, 0.0017971238510697952, 0.001824766783448256, 0.0018273914436611356, 0.0018233456662710829, 0.001811169776658133, 0.001808649772361402, 0.0017980740166243004, 0.0017838545825434003, 0.001763256645783561, 0.0017210445082360198, 0.001701132343137258, 0.0016754062664861471, 0.001664623953019805, 0.0016487024832499652, 0.0016273141189128994, 0.0016010950578146683, 0.0015728930425157306, 0.0015352912734848325, 0.0015149109108664593, 0.001483448037548582, 0.0014523514599372237, 0.0014315579818603703, 0.0014274984339550348, 0.0014181675327994876, 0.0014143999198181453, 0.0014053113797315735, 0.0013993515007172275, 0.001408693418285001, 0.0013985390403155494, 0.001397974449188959, 0.0013917694550025816, 0.0013787315311329358, 0.0013626448151797038, 0.0013449083914956062, 0.0013370509354753064, 0.001325880293477993, 0.0013185543793476045, 0.001294420174263172, 0.00127875483607759, 0.0012659041912157889, 0.0012433398248735822, 0.001228894554342046, 0.0012003400138518715, 0.001183988904005212, 0.0011747543964566436, 0.0011585547622780935, 0.0011605046672421217, 0.0011473565792502146, 0.0011370039058606926, 0.0011340652778993677, 0.0011226770617605876, 0.0011216442731143861, 0.0011107600578349525, 0.0011026409620242816, 0.0010866919512238764, 0.0010731362559796018, 0.001051089661012024, 0.0010301832647098524, 0.001009888279286232, 0.0009965887156262153, 0.0009909235256389188, 0.0009767536654130364, 0.0009747817276245561, 0.0009568910741692924, 0.000949947980363763, 0.000956703795161448, 0.0009593917997446279, 0.0009746082191319944, 0.0009815127554947322, 0.0009862085012061277, 0.0009848589907084247, 0.0009587748806599638, 0.0009397330121270677, 0.0009244532483694009, 0.0009160174307072283, 0.0009138141482619988, 0.0009141501488348964, 0.0009184162544694721, 0.0009130457535092251, 0.000912208506180038, 0.0009004897976744733, 0.0008954966088329721, 0.000888658170943591, 0.000878327530378521, 0.0008779392018475493, 0.0008724833236925496, 0.0008753007711193868, 0.0008733894235981503, 0.0008842763929806406, 0.0008803270091975667, 0.0008834474079606231, 0.0008812331091031674, 0.0008784927765619131, 0.0008838109495640858, 0.0008909550928927427, 0.000899184352825675, 0.0009081654828930417, 0.000914194214483801, 0.0009259542345352136, 0.0009387635678511666, 0.0009425339349355657, 0.0009425063939050002, 0.0009326494590656548, 0.0009267529244216092, 0.0009192645182108854, 0.0009126023429171226, 0.0009054058716303917, 0.0008956756255316468, 0.0008975015958581308, 0.0008902445343041561, 0.0008840973762819658, 0.0008824283898297043, 0.0008799772381093866, 0.000884678492026895, 0.0008933897199947213, 0.0008983829088362226, 0.000893860671617389, 0.0008973749071175302, 0.0009013435696219998, 0.0009055848883290665, 0.0009138995254567515, 0.0009202174378684471, 0.000930589389979365, 0.000922150818214136, 0.0009280666315795773, 0.0009267253833910438, 0.0009243623629685353, 0.0009317653919845064, 0.0009418922289233926, 0.0009494384712983037, 0.0009643051195974898, 0.0009718458537662879, 0.0009862966325039368, 0.0009917001827008621, 0.0009979795376697665, 0.001014038712592433, 0.0010172830459930335, 0.0010330585483008768, 0.0010469640146333317, 0.001060098332109956, 0.0010826544361429932, 0.0011030761103072145, 0.0011350760337211167, 0.0011531154087414334, 0.0011576624328877758, 0.0011768364983673857, 0.0011841624124977737, 0.0011999406689086737, 0.0012165093528967996, 0.0012281895039595726, 0.0012561601746017613, 0.0012707651831105765, 0.001307240523991351, 0.001333627585376031, 0.0013666217399933432, 0.0014024911782016796, 0.0014332324765187446, 0.0014678102403935655, 0.0014988241949132272, 0.0015329365153714935, 0.0015343879276822883, 0.0015720971067323913, 0.0016118636007657278, 0.001651087536496926, 0.0016970920739533186, 0.001745473402347502, 0.0017665615694514051, 0.0018051024876245825, 0.0018256783915599696, 0.0018815618966801597, 0.0018972630382054765, 0.0019475088943689358, 0.001967589059754146, 0.0019944801219981727, 0.0020293085092511383, 0.0020797967264835726, 0.002127649267090901, 0.002177592171918141, 0.002209096356781867, 0.0022576126362258207, 0.0022860239633570555, 0.002367479315357191, 0.00239798651491445, 0.002459918030346795, 0.002492961758819125, 0.0025305745442622493, 0.0025619850896220525, 0.0025918974029190997, 0.0026126908809959533, 0.0026649499864937407, 0.002671884817990101, 0.0027487573425041584, 0.0027664331759210126, 0.0028080311484869457, 0.002835572179052315, 0.002897776350687257, 0.0029281981730497637, 0.0029626547563900967, 0.002993387792397992, 0.0030170785868903222, 0.0030149964849795806, 0.0030319039236436605, 0.0030360240618162396, 0.0030334957952103388, 0.0030378693108641195, 0.003026379192912247, 0.0030242502712495446, 0.0030348563221202682, 0.0030418489897808152, 0.0030719182869520852, 0.0030982750532031434, 0.0030908086798168716, 0.0031010319103627363, 0.0031036813575031253, 0.0030762670156783568, 0.003066933360419753, 0.003042223547796504, 0.0030263378813663996, 0.003004663090311454, 0.0029920548065186284, 0.0029706664421815625, 0.0029578268137319874, 0.0029413352446294445, 0.0029132489016588815, 0.0028961762168114094, 0.002857943758180564, 0.00283680050901553, 0.0028030104186148787, 0.0027938640423641197, 0.0027516161014768444, 0.002719478472910115, 0.0026733913123620267, 0.002627637398283779, 0.0025728335015617514, 0.0025436510255746865, 0.002504355483164018, 0.0024615594757684913, 0.002436053727361903, 0.0024182842544411267, 0.0024007185851465346, 0.0023905779776923655, 0.0023550968680150007, 0.002333292634116398, 0.002292746728918062, 0.0022553735504408563, 0.0022384468330553806, 0.002203128215458351, 0.00217902430550754, 0.002143711196116624, 0.0021122262899742946, 0.0020506142504965077, 0.00203825383597877, 0.0020262487007553258, 0.0020074629638066875, 0.0019932738248594093, 0.0019544327094530695, 0.0019488088310116213, 0.0019049882972790627, 0.0018915620448784454, 0.0018528393559035367, 0.001821197465886984, 0.0017890212798774634, 0.0017354539754278208, 0.0016897689139259869, 0.001663423164087155, 0.0016456371665480398, 0.0016412085688331283, 0.001628644350689207, 0.0016130809143167168, 0.0016073331012377244, 0.001603339651805746, 0.0015941712427305346, 0.001588935692820058, 0.0015824029603699523, 0.00157714813173808, 0.0015643332902160138, 0.0015630746651191763, 0.0015527274999357675, 0.0015555421932595482, 0.0015637163711313498, 0.0015732180266764021, 0.001592557338339404, 0.001584653062567143, 0.0015960522951181493, 0.0016165015103129358, 0.0016268707083207973, 0.0016398039762742945, 0.001641899848700319, 0.0016484215647381982, 0.0016487190078683044, 0.0016555629539637985, 0.0016557612493838694, 0.0016741145921526312, 0.0017004658501975761, 0.0017330110860166727, 0.0017605190673453631, 0.0017664348807108045, 0.0017779084740443371, 0.001790398331405732, 0.0018131775177863488, 0.0018366452299310996, 0.0018605453362557267, 0.0018882543671075445, 0.0018984252696953353, 0.001914192509694009, 0.0019416316384462862, 0.0019781785860065308, 0.0020108477564631713, 0.0020298097560074277, 0.0020661143424986973, 0.002068810609391047, 0.002110609631480107, 0.002115869968318093, 0.0021256800834054774, 0.0021556667574850513, 0.002178443189762611, 0.0021840174943490416, 0.002213334921385877, 0.002212183706308245, 0.00223874152208243, 0.0022391546375409104, 0.002258397555596934, 0.0022739802706908193, 0.0023094503639559585, 0.002319709397841558, 0.002351866305129683, 0.002368812301236555, 0.0023749456887434623, 0.002389630566240917, 0.0023986777947816403, 0.00241149814450982, 0.0024190003212358263, 0.0024229882624616918, 0.002422095933071374, 0.002423731870286957, 0.0024201625527256847, 0.0024417767535133868, 0.0024415812121963724, 0.002455808908586442, 0.002457513698378438, 0.0024465385976981386, 0.0024522313287160006, 0.0024169705472831585, 0.0024148361174143426, 0.0023995701241719585, 0.0023793853028705996, 0.0023548297200185167, 0.002332361747283289, 0.0023205108418310103, 0.0022940521737668603, 0.0022523164960481005, 0.0022274744864781374, 0.0022039158889325208, 0.0021684926154193433, 0.0021411526343771015, 0.002118635087786856, 0.002083801192327777, 0.002047124801923875, 0.0020278653592495127, 0.0019697703093749233, 0.0019519264756716211, 0.0019212622922401392, 0.0018812286502103187, 0.0018427428140982722, 0.001812265909674635, 0.00175640994558501, 0.0017214080498394828, 0.0016736711815605288, 0.0016349457384825634, 0.0015946835058990505, 0.0015675610989982752, 0.0015259052902681545, 0.0014996366553149056, 0.001476708747369236, 0.001439175830914751, 0.0014011692087345419, 0.0013630882257718063, 0.0013162216540587178, 0.0012905451512626243, 0.0012539458757443056, 0.0012235736272368167, 0.0012001196856073486, 0.001185272316029558, 0.0011544346241055146, 0.0011379100057662933, 0.0010844501113358553, 0.0010647610285846733, 0.0010130802847287583, 0.0009929670701068693, 0.0009656849252288149, 0.0009476042386626501, 0.0009280005331062204, 0.0009123489654359212, 0.0008921173243826012, 0.0008740696870531149, 0.000861342976828858, 0.0008399518583887359, 0.0008269304591374295, 0.000805963472568014, 0.0007840931401960546, 0.0007730684656607372, 0.0007618757908389714, 0.000755502796366145, 0.0007484440302322409, 0.0007361304354664644, 0.0007236515945172958, 0.0007035631668229157, 0.0006909796699575985, 0.0006775396470416985, 0.0006603843391025302, 0.0006506954045496334, 0.0006404831904159946, 0.0006315406177914192, 0.000626814576946402, 0.0006201799426832045, 0.0006156053775062967, 0.0006078663479174281, 0.0005998298751984535, 0.0005900335306263518, 0.0005812644664943382, 0.0005748804556092857, 0.0005698349388097101, 0.000566761359798615, 0.0005616442363195694, 0.0005622749259195163, 0.0005532993040582626, 0.0005422911541412846, 0.0005348495676825219, 0.0005325361211150309, 0.0005320376284617976, 0.0005307018884793774, 0.0005264054877111798, 0.0005264054877111798, 0.0005228637111804734, 0.0005181238998201733, 0.0005176309153730532, 0.0005136154331166225, 0.0005124091359778592, 0.0005101562796776121, 0.0005055431570579128, 0.0004995529829099451, 0.0004920150028442035, 0.0004884759804165536, 0.00048560345092858563, 0.000481450263519328, 0.000479029406932632, 0.00047415189041950524, 0.00047243608421528277, 0.0004715299843096821, 0.00047353772543789753, 0.00047000971942247376, 0.0004698554896513077, 0.0004721276246729506, 0.0004682388311571205, 0.0004696351614067847, 0.0004644106279085342, 0.00046173088563452376, 0.0004594807834373332, 0.0004550053659704607, 0.0004509155229315034, 0.00044808430498938354, 0.0004430277717775818, 0.0004410696045043841, 0.00043787759906185783, 0.00043347929648056836, 0.0004299017166101269, 0.00042542354504019795, 0.00042215993291820175, 0.00041868425486085215, 0.000416883071461877, 0.0004110388647759057, 0.0004118981449295452, 0.00040788541677617095, 0.00040867033614728403, 0.00040761000647051725, 0.0004041866563712419, 0.00040178507850594175, 0.00039903372955246133, 0.0003977007436730975, 0.0003977310388067194, 0.00039884645054461687, 0.00039690480788975835, 0.000394671230310907, 0.0003933712936682215, 0.00039117076532604856, 0.0003899947633209073, 0.00038895095826247983, 0.00038990112381698505, 0.00038822662915861066, 0.0003852577060636639, 0.00038354740806555447, 0.0003831673418437523, 0.00038108523993301045, 0.00038199133983861106, 0.0003807712721845652, 0.0003789921216100424, 0.0003772350038599718, 0.00037759028315426514, 0.0003756155912627282, 0.0003736216206497954, 0.000373136898511845, 0.0003710079768491419, 0.0003707132878220925, 0.0003699917128212798, 0.00036924259678990177, 0.0003697686304737003, 0.000369484957858877, 0.0003692976788510325, 0.00037006056539769325, 0.00036974108944313496, 0.00036845492331573224, 0.0003671825277036122, 0.0003674441674939832, 0.00036729820003198675, 0.00036671708428705744, 0.0003670723635813507, 0.0003662516408705027, 0.0003653593114801848, 0.0003654336722627113, 0.00036621859163382426, 0.0003649076385789127, 0.0003645000313265452, 0.00036404009611610357, 0.00036481399907499045, 0.00036354435756592694, 0.0003624454704463687, 0.00036318632416857717, 0.000362616224835874, 0.00036201858447260554, 0.0003629026515537539, 0.00036316429134412485, 0.0003618092726403087, 0.00036178173160974337, 0.0003609059268377646, 0.0003606580575626763, 0.00035972441662651027, 0.00035978776099681063, 0.0003598290725426587, 0.0003593278257863689, 0.00035902487445014993, 0.0003587962838964574, 0.00035836939792269413, 0.00035583837721373673, 0.0003554059830338604, 0.0003547532606094612, 0.0003549102444836838, 0.00035429057129596295, 0.0003543126041204152, 0.0003549185067928534, 0.0003548248672889311, 0.00035513057272820676, 0.0003544998831282598, 0.00035434014515098067, 0.000354516407746599, 0.00035333489753534467, 0.0003535855209134895, 0.0003530154215807864, 0.0003527152243476239, 0.0003532798154742139, 0.00035263260125592777, 0.0003519964034498677, 0.000351608074918896, 0.00035093882787615757, 0.000349443349916458, 0.00034942957940117537, 0.0003491624314046913, 0.00034956453045094566, 0.00034901095573658175, 0.00034910184113744744, 0.0003489310867479422, 0.0003488181685226241, 0.0003479836752964935, 0.0003476917403725006, 0.00034843259409470895, 0.0003489586277785075, 0.0003480910853156984, 0.0003474548875096384, 0.0003469619030625183, 0.00034665344352018617, 0.0003463918037298151, 0.00034654052529486815, 0.00034605304905386115, 0.0003454196053508576, 0.00034516347376659963, 0.00034559862204953256, 0.0003448357355028718, 0.0003449403914190202, 0.00034430419361296017, 0.00034424635744877293, 0.000344852260121211, 0.0003448384896059283, 0.0003451028834993559, 0.0003437423565894266, 0.0003425580922751158, 0.00034259664971790727, 0.0003416354677511759, 0.00034174838597649394, 0.00034173461546121124, 0.0003417869434192854, 0.0003409965158420593, 0.00034094143378092864, 0.0003408477942770064, 0.0003402501539137379, 0.0003404980231888262, 0.0003398783500011054, 0.00033904936498108774, 0.00033842969179336696, 0.00033828372433137053, 0.0003380661501899041, 0.00033740791955939176, 0.000338358085113897, 0.0003377081167925543, 0.00033727847671573453, 0.000337388640837996, 0.00033701959102842003, 0.00033749605085720095, 0.00033774116602923275, 0.0003364384752834908, 0.000335931720321088, 0.0003357031297673954, 0.00033592070390886183, 0.0003353395881639325, 0.00033492922680850853, 0.00033513303043469225, 0.00033468961984258985, 0.0003348713906443213, 0.00033494024322073466, 0.0003348108003770775, 0.00033487689885043436, 0.00033441145543387964, 0.0003341993894985263, 0.0003345464064836499, 0.00033424896335354395, 0.00033390194636842026, 0.00033334837165405635, 0.00033337040447850867, 0.0003331583385431553, 0.0003329132233711235, 0.0003332326993256818, 0.0003335301424557878, 0.0003335026014252224, 0.00033401761869679484, 0.0003333428634479433, 0.00033282509207331433, 0.00033313630571870306, 0.0003330839777606288, 0.00033270666564188324, 0.00033214758272140626, 0.00033204843501137094, 0.00033124974512497527, 0.0003311781384455053, 0.00033189695934326144, 0.0003313213518044452, 0.0003320980088663886, 0.0003318336149729611, 0.00033207873014499283, 0.0003325304030462649, 0.0003314094831022544, 0.00033175650008737803]]
  in  "Stop":bool
  out "Picture":cluster{dbl[], dbl[]}[](graph)
  in  "Start Measurement":bool
  out "CCD IMAGE":dbl[][](graph)
  in  "Arc length (deg)":dbl=90.0
  in  "Angle step (deg)":dbl=1.0
  in  "Center angle (deg)":dbl=90.0
  in  "Radial step":dbl=1.0
  in  "Visible":bool=TRUE
  in  "Inner radius":dbl(slide) scale=0.0..1.0
  in  "Outer radius":dbl(slide)=0.9325842696629213 scale=0.0..1.0
  in  "Path":string="E:\\Data\\Data Rabitt\\"
  in  "Name":string="image"
  in  "Index":i32=1
  in  "Run Scan":bool
  in  "Analyze":bool
  in  "Save image":bool
  in  "Start Delay (fs)":dbl format="%.3f"
  out "Current Delay (fs)":dbl
  out "Actual delay  (fs)":dbl=inf format="%.3f"
  in  "Angle":dbl min=0.0 max=5.0 format="%.3f"
  in  "Delay Stage Move":bool
  in  "Step (fs)":dbl=0.13 format="%.3f"
  in  "Max Steps":i32=60
  out "StepNb":i32
  out "Angle [deg]":ext(graph)
  out "Nb of shot":i32
  out "XUV":dbl[][](graph)=[[0.0010313840536425023, 0.0010313840536425023, 0.0010274759814052766, 0.0010401531177745159, 0.00104452387932524, 0.0010522711712232782, 0.001047206375702307, 0.0010453914217880493, 0.0010393489196820073, 0.0010272942106035452, 0.0010408196107141979, 0.0010468510964080136, 0.001062026204249532, 0.001106433361933133, 0.001154520001300267, 0.0011934960677563772, 0.001214033414248973, 0.0012241024150236718, 0.0012391453259184763, 0.0012555680424446059, 0.0012925281054633312, 0.001352528994653044, 0.0014089853532089937, 0.0014660421062312687, 0.0015363130457188075, 0.0015691474623588406, 0.0016108363203256395, 0.0016140062929437132, 0.0015863330654316305, 0.001566139981821102, 0.0015480455247396548, 0.0015630250912641588, 0.0016089194645982896, 0.0016388896140595243, 0.0016752961023638853, 0.001688323009821305, 0.0016919033437948032, 0.0017147706614732288, 0.0017464097973867246, 0.001779717919752482, 0.001837171263614898, 0.00188523587015758, 0.001909243386501412, 0.0019293676175355272, 0.0019505631946586353, 0.0019533283141273984, 0.001977616748982997, 0.0019911972311547808, 0.002017708227177005, 0.002053718124641225, 0.0020883013967221585, 0.002112669700566397, 0.0021315656016372966, 0.0021208218456137463, 0.002105299720787104, 0.002099830072116822, 0.0021012126318512036, 0.0020908214010188896, 0.002095054457416787, 0.002100080695494967, 0.0021084586769929523, 0.0020993728910094368, 0.002104955457905037, 0.0020792872174181134, 0.0020928346503532183, 0.0020942117018814864, 0.002102964241395161, 0.0021093372358679877, 0.002121036665652156, 0.002136567052787968, 0.002154127213876447, 0.002169360157882152, 0.0021869395976920275, 0.0021825908689657556, 0.002171045668952753, 0.0021674267775364637, 0.0021489908116760054, 0.002157660728097984, 0.002145658346977596, 0.002135917084466625, 0.00209696855904108, 0.0020850653256307278, 0.0020535996982097935, 0.002049595232365589, 0.0020524236962046524, 0.0020767176392663643, 0.002111884781195284, 0.002137809153266466, 0.0021668842192343256, 0.00216397037820051, 0.0021656008072099796, 0.0021352698702483386, 0.0021013916485498785, 0.0020823029602650214, 0.0020479290000163844, 0.0020333460243320213, 0.0020002169186649392, 0.0019659586307446764, 0.0019358700548520106, 0.0019274369912928948, 0.0019173046461478957, 0.001900014387158957, 0.0018599917615413628, 0.001814549061108504, 0.0017608991335671654, 0.0017321325271416374, 0.0017011240808280886, 0.0016809695546603515, 0.0016804848325224012, 0.001677022924980334, 0.0016912533754734602, 0.0016999535870290603, 0.0017145172839920274, 0.001701024933118053, 0.0017087557003977521, 0.0017038864461937952, 0.0017154509249281934, 0.0017378638156022909, 0.001773105318313737, 0.0017971238510697952, 0.001824766783448256, 0.0018273914436611356, 0.0018233456662710829, 0.001811169776658133, 0.001808649772361402, 0.0017980740166243004, 0.0017838545825434003, 0.001763256645783561, 0.0017210445082360198, 0.001701132343137258, 0.0016754062664861471, 0.001664623953019805, 0.0016487024832499652, 0.0016273141189128994, 0.0016010950578146683, 0.0015728930425157306, 0.0015352912734848325, 0.0015149109108664593, 0.001483448037548582, 0.0014523514599372237, 0.0014315579818603703, 0.0014274984339550348, 0.0014181675327994876, 0.0014143999198181453, 0.0014053113797315735, 0.0013993515007172275, 0.001408693418285001, 0.0013985390403155494, 0.001397974449188959, 0.0013917694550025816, 0.0013787315311329358, 0.0013626448151797038, 0.0013449083914956062, 0.0013370509354753064, 0.001325880293477993, 0.0013185543793476045, 0.001294420174263172, 0.00127875483607759, 0.0012659041912157889, 0.0012433398248735822, 0.001228894554342046, 0.0012003400138518715, 0.001183988904005212, 0.0011747543964566436, 0.0011585547622780935, 0.0011605046672421217, 0.0011473565792502146, 0.0011370039058606926, 0.0011340652778993677, 0.0011226770617605876, 0.0011216442731143861, 0.0011107600578349525, 0.0011026409620242816, 0.0010866919512238764, 0.0010731362559796018, 0.001051089661012024, 0.0010301832647098524, 0.001009888279286232, 0.0009965887156262153, 0.0009909235256389188, 0.0009767536654130364, 0.0009747817276245561, 0.0009568910741692924, 0.000949947980363763, 0.000956703795161448, 0.0009593917997446279, 0.0009746082191319944, 0.0009815127554947322, 0.0009862085012061277, 0.0009848589907084247, 0.0009587748806599638, 0.0009397330121270677, 0.0009244532483694009, 0.0009160174307072283, 0.0009138141482619988, 0.0009141501488348964, 0.0009184162544694721, 0.0009130457535092251, 0.000912208506180038, 0.0009004897976744733, 0.0008954966088329721, 0.000888658170943591, 0.000878327530378521, 0.0008779392018475493, 0.0008724833236925496, 0.0008753007711193868, 0.0008733894235981503, 0.0008842763929806406, 0.0008803270091975667, 0.0008834474079606231, 0.0008812331091031674, 0.0008784927765619131, 0.0008838109495640858, 0.0008909550928927427, 0.000899184352825675, 0.0009081654828930417, 0.000914194214483801, 0.0009259542345352136, 0.0009387635678511666, 0.0009425339349355657, 0.0009425063939050002, 0.0009326494590656548, 0.0009267529244216092, 0.0009192645182108854, 0.0009126023429171226, 0.0009054058716303917, 0.0008956756255316468, 0.0008975015958581308, 0.0008902445343041561, 0.0008840973762819658, 0.0008824283898297043, 0.0008799772381093866, 0.000884678492026895, 0.0008933897199947213, 0.0008983829088362226, 0.000893860671617389, 0.0008973749071175302, 0.0009013435696219998, 0.0009055848883290665, 0.0009138995254567515, 0.0009202174378684471, 0.000930589389979365, 0.000922150818214136, 0.0009280666315795773, 0.0009267253833910438, 0.0009243623629685353, 0.0009317653919845064, 0.0009418922289233926, 0.0009494384712983037, 0.0009643051195974898, 0.0009718458537662879, 0.0009862966325039368, 0.0009917001827008621, 0.0009979795376697665, 0.001014038712592433, 0.0010172830459930335, 0.0010330585483008768, 0.0010469640146333317, 0.001060098332109956, 0.0010826544361429932, 0.0011030761103072145, 0.0011350760337211167, 0.0011531154087414334, 0.0011576624328877758, 0.0011768364983673857, 0.0011841624124977737, 0.0011999406689086737, 0.0012165093528967996, 0.0012281895039595726, 0.0012561601746017613, 0.0012707651831105765, 0.001307240523991351, 0.001333627585376031, 0.0013666217399933432, 0.0014024911782016796, 0.0014332324765187446, 0.0014678102403935655, 0.0014988241949132272, 0.0015329365153714935, 0.0015343879276822883, 0.0015720971067323913, 0.0016118636007657278, 0.001651087536496926, 0.0016970920739533186, 0.001745473402347502, 0.0017665615694514051, 0.0018051024876245825, 0.0018256783915599696, 0.0018815618966801597, 0.0018972630382054765, 0.0019475088943689358, 0.001967589059754146, 0.0019944801219981727, 0.0020293085092511383, 0.0020797967264835726, 0.002127649267090901, 0.002177592171918141, 0.002209096356781867, 0.0022576126362258207, 0.0022860239633570555, 0.002367479315357191, 0.00239798651491445, 0.002459918030346795, 0.002492961758819125, 0.0025305745442622493, 0.0025619850896220525, 0.0025918974029190997, 0.0026126908809959533, 0.0026649499864937407, 0.002671884817990101, 0.0027487573425041584, 0.0027664331759210126, 0.0028080311484869457, 0.002835572179052315, 0.002897776350687257, 0.0029281981730497637, 0.0029626547563900967, 0.002993387792397992, 0.0030170785868903222, 0.0030149964849795806, 0.0030319039236436605, 0.0030360240618162396, 0.0030334957952103388, 0.0030378693108641195, 0.003026379192912247, 0.0030242502712495446, 0.0030348563221202682, 0.0030418489897808152, 0.0030719182869520852, 0.0030982750532031434, 0.0030908086798168716, 0.0031010319103627363, 0.0031036813575031253, 0.0030762670156783568, 0.003066933360419753, 0.003042223547796504, 0.0030263378813663996, 0.003004663090311454, 0.0029920548065186284, 0.0029706664421815625, 0.0029578268137319874, 0.0029413352446294445, 0.0029132489016588815, 0.0028961762168114094, 0.002857943758180564, 0.00283680050901553, 0.0028030104186148787, 0.0027938640423641197, 0.0027516161014768444, 0.002719478472910115, 0.0026733913123620267, 0.002627637398283779, 0.0025728335015617514, 0.0025436510255746865, 0.002504355483164018, 0.0024615594757684913, 0.002436053727361903, 0.0024182842544411267, 0.0024007185851465346, 0.0023905779776923655, 0.0023550968680150007, 0.002333292634116398, 0.002292746728918062, 0.0022553735504408563, 0.0022384468330553806, 0.002203128215458351, 0.00217902430550754, 0.002143711196116624, 0.0021122262899742946, 0.0020506142504965077, 0.00203825383597877, 0.0020262487007553258, 0.0020074629638066875, 0.0019932738248594093, 0.0019544327094530695, 0.0019488088310116213, 0.0019049882972790627, 0.0018915620448784454, 0.0018528393559035367, 0.001821197465886984, 0.0017890212798774634, 0.0017354539754278208, 0.0016897689139259869, 0.001663423164087155, 0.0016456371665480398, 0.0016412085688331283, 0.001628644350689207, 0.0016130809143167168, 0.0016073331012377244, 0.001603339651805746, 0.0015941712427305346, 0.001588935692820058, 0.0015824029603699523, 0.00157714813173808, 0.0015643332902160138, 0.0015630746651191763, 0.0015527274999357675, 0.0015555421932595482, 0.0015637163711313498, 0.0015732180266764021, 0.001592557338339404, 0.001584653062567143, 0.0015960522951181493, 0.0016165015103129358, 0.0016268707083207973, 0.0016398039762742945, 0.001641899848700319, 0.0016484215647381982, 0.0016487190078683044, 0.0016555629539637985, 0.0016557612493838694, 0.0016741145921526312, 0.0017004658501975761, 0.0017330110860166727, 0.0017605190673453631, 0.0017664348807108045, 0.0017779084740443371, 0.001790398331405732, 0.0018131775177863488, 0.0018366452299310996, 0.0018605453362557267, 0.0018882543671075445, 0.0018984252696953353, 0.001914192509694009, 0.0019416316384462862, 0.0019781785860065308, 0.0020108477564631713, 0.0020298097560074277, 0.0020661143424986973, 0.002068810609391047, 0.002110609631480107, 0.002115869968318093, 0.0021256800834054774, 0.0021556667574850513, 0.002178443189762611, 0.0021840174943490416, 0.002213334921385877, 0.002212183706308245, 0.00223874152208243, 0.0022391546375409104, 0.002258397555596934, 0.0022739802706908193, 0.0023094503639559585, 0.002319709397841558, 0.002351866305129683, 0.002368812301236555, 0.0023749456887434623, 0.002389630566240917, 0.0023986777947816403, 0.00241149814450982, 0.0024190003212358263, 0.0024229882624616918, 0.002422095933071374, 0.002423731870286957, 0.0024201625527256847, 0.0024417767535133868, 0.0024415812121963724, 0.002455808908586442, 0.002457513698378438, 0.0024465385976981386, 0.0024522313287160006, 0.0024169705472831585, 0.0024148361174143426, 0.0023995701241719585, 0.0023793853028705996, 0.0023548297200185167, 0.002332361747283289, 0.0023205108418310103, 0.0022940521737668603, 0.0022523164960481005, 0.0022274744864781374, 0.0022039158889325208, 0.0021684926154193433, 0.0021411526343771015, 0.002118635087786856, 0.002083801192327777, 0.002047124801923875, 0.0020278653592495127, 0.0019697703093749233, 0.0019519264756716211, 0.0019212622922401392, 0.0018812286502103187, 0.0018427428140982722, 0.001812265909674635, 0.00175640994558501, 0.0017214080498394828, 0.0016736711815605288, 0.0016349457384825634, 0.0015946835058990505, 0.0015675610989982752, 0.0015259052902681545, 0.0014996366553149056, 0.001476708747369236, 0.001439175830914751, 0.0014011692087345419, 0.0013630882257718063, 0.0013162216540587178, 0.0012905451512626243, 0.0012539458757443056, 0.0012235736272368167, 0.0012001196856073486, 0.001185272316029558, 0.0011544346241055146, 0.0011379100057662933, 0.0010844501113358553, 0.0010647610285846733, 0.0010130802847287583, 0.0009929670701068693, 0.0009656849252288149, 0.0009476042386626501, 0.0009280005331062204, 0.0009123489654359212, 0.0008921173243826012, 0.0008740696870531149, 0.000861342976828858, 0.0008399518583887359, 0.0008269304591374295, 0.000805963472568014, 0.0007840931401960546, 0.0007730684656607372, 0.0007618757908389714, 0.000755502796366145, 0.0007484440302322409, 0.0007361304354664644, 0.0007236515945172958, 0.0007035631668229157, 0.0006909796699575985, 0.0006775396470416985, 0.0006603843391025302, 0.0006506954045496334, 0.0006404831904159946, 0.0006315406177914192, 0.000626814576946402, 0.0006201799426832045, 0.0006156053775062967, 0.0006078663479174281, 0.0005998298751984535, 0.0005900335306263518, 0.0005812644664943382, 0.0005748804556092857, 0.0005698349388097101, 0.000566761359798615, 0.0005616442363195694, 0.0005622749259195163, 0.0005532993040582626, 0.0005422911541412846, 0.0005348495676825219, 0.0005325361211150309, 0.0005320376284617976, 0.0005307018884793774, 0.0005264054877111798, 0.0005264054877111798, 0.0005228637111804734, 0.0005181238998201733, 0.0005176309153730532, 0.0005136154331166225, 0.0005124091359778592, 0.0005101562796776121, 0.0005055431570579128, 0.0004995529829099451, 0.0004920150028442035, 0.0004884759804165536, 0.00048560345092858563, 0.000481450263519328, 0.000479029406932632, 0.00047415189041950524, 0.00047243608421528277, 0.0004715299843096821, 0.00047353772543789753, 0.00047000971942247376, 0.0004698554896513077, 0.0004721276246729506, 0.0004682388311571205, 0.0004696351614067847, 0.0004644106279085342, 0.00046173088563452376, 0.0004594807834373332, 0.0004550053659704607, 0.0004509155229315034, 0.00044808430498938354, 0.0004430277717775818, 0.0004410696045043841, 0.00043787759906185783, 0.00043347929648056836, 0.0004299017166101269, 0.00042542354504019795, 0.00042215993291820175, 0.00041868425486085215, 0.000416883071461877, 0.0004110388647759057, 0.0004118981449295452, 0.00040788541677617095, 0.00040867033614728403, 0.00040761000647051725, 0.0004041866563712419, 0.00040178507850594175, 0.00039903372955246133, 0.0003977007436730975, 0.0003977310388067194, 0.00039884645054461687, 0.00039690480788975835, 0.000394671230310907, 0.0003933712936682215, 0.00039117076532604856, 0.0003899947633209073, 0.00038895095826247983, 0.00038990112381698505, 0.00038822662915861066, 0.0003852577060636639, 0.00038354740806555447, 0.0003831673418437523, 0.00038108523993301045, 0.00038199133983861106, 0.0003807712721845652, 0.0003789921216100424, 0.0003772350038599718, 0.00037759028315426514, 0.0003756155912627282, 0.0003736216206497954, 0.000373136898511845, 0.0003710079768491419, 0.0003707132878220925, 0.0003699917128212798, 0.00036924259678990177, 0.0003697686304737003, 0.000369484957858877, 0.0003692976788510325, 0.00037006056539769325, 0.00036974108944313496, 0.00036845492331573224, 0.0003671825277036122, 0.0003674441674939832, 0.00036729820003198675, 0.00036671708428705744, 0.0003670723635813507, 0.0003662516408705027, 0.0003653593114801848, 0.0003654336722627113, 0.00036621859163382426, 0.0003649076385789127, 0.0003645000313265452, 0.00036404009611610357, 0.00036481399907499045, 0.00036354435756592694, 0.0003624454704463687, 0.00036318632416857717, 0.000362616224835874, 0.00036201858447260554, 0.0003629026515537539, 0.00036316429134412485, 0.0003618092726403087, 0.00036178173160974337, 0.0003609059268377646, 0.0003606580575626763, 0.00035972441662651027, 0.00035978776099681063, 0.0003598290725426587, 0.0003593278257863689, 0.00035902487445014993, 0.0003587962838964574, 0.00035836939792269413, 0.00035583837721373673, 0.0003554059830338604, 0.0003547532606094612, 0.0003549102444836838, 0.00035429057129596295, 0.0003543126041204152, 0.0003549185067928534, 0.0003548248672889311, 0.00035513057272820676, 0.0003544998831282598, 0.00035434014515098067, 0.000354516407746599, 0.00035333489753534467, 0.0003535855209134895, 0.0003530154215807864, 0.0003527152243476239, 0.0003532798154742139, 0.00035263260125592777, 0.0003519964034498677, 0.000351608074918896, 0.00035093882787615757, 0.000349443349916458, 0.00034942957940117537, 0.0003491624314046913, 0.00034956453045094566, 0.00034901095573658175, 0.00034910184113744744, 0.0003489310867479422, 0.0003488181685226241, 0.0003479836752964935, 0.0003476917403725006, 0.00034843259409470895, 0.0003489586277785075, 0.0003480910853156984, 0.0003474548875096384, 0.0003469619030625183, 0.00034665344352018617, 0.0003463918037298151, 0.00034654052529486815, 0.00034605304905386115, 0.0003454196053508576, 0.00034516347376659963, 0.00034559862204953256, 0.0003448357355028718, 0.0003449403914190202, 0.00034430419361296017, 0.00034424635744877293, 0.000344852260121211, 0.0003448384896059283, 0.0003451028834993559, 0.0003437423565894266, 0.0003425580922751158, 0.00034259664971790727, 0.0003416354677511759, 0.00034174838597649394, 0.00034173461546121124, 0.0003417869434192854, 0.0003409965158420593, 0.00034094143378092864, 0.0003408477942770064, 0.0003402501539137379, 0.0003404980231888262, 0.0003398783500011054, 0.00033904936498108774, 0.00033842969179336696, 0.00033828372433137053, 0.0003380661501899041, 0.00033740791955939176, 0.000338358085113897, 0.0003377081167925543, 0.00033727847671573453, 0.000337388640837996, 0.00033701959102842003, 0.00033749605085720095, 0.00033774116602923275, 0.0003364384752834908, 0.000335931720321088, 0.0003357031297673954, 0.00033592070390886183, 0.0003353395881639325, 0.00033492922680850853, 0.00033513303043469225, 0.00033468961984258985, 0.0003348713906443213, 0.00033494024322073466, 0.0003348108003770775, 0.00033487689885043436, 0.00033441145543387964, 0.0003341993894985263, 0.0003345464064836499, 0.00033424896335354395, 0.00033390194636842026, 0.00033334837165405635, 0.00033337040447850867, 0.0003331583385431553, 0.0003329132233711235, 0.0003332326993256818, 0.0003335301424557878, 0.0003335026014252224, 0.00033401761869679484, 0.0003333428634479433, 0.00033282509207331433, 0.00033313630571870306, 0.0003330839777606288, 0.00033270666564188324, 0.00033214758272140626, 0.00033204843501137094, 0.00033124974512497527, 0.0003311781384455053, 0.00033189695934326144, 0.0003313213518044452, 0.0003320980088663886, 0.0003318336149729611, 0.00033207873014499283, 0.0003325304030462649, 0.0003314094831022544, 0.00033175650008737803]]
  out "Camera Status:":bool
  out "Raw Image":i32[][](graph)
  out "VBI":i32[](graph)
  in  "Tab Control 2":enum32{"Camera Cursor", "Harmonics"}(tab)
  in  "Calibration Date":u16(ring) items=["first calibration - 7/31", "7/31-current"]
  in  "Laser:":u16(ring) items=["800nm  "]
  in  "Grating:":u16(ring) items=["Shimadzu 30-006  "]
  out "Distance to nearest harmonic of 800nm (pixels)":dbl
  out "Cursor Position (pixels)":dbl
  out "Nearest Harmonic of 800nm":dbl
  out "E (eV)":dbl
  out "E (J)":dbl
  out "l (nm)":dbl
  in  "Harmonic":dbl min=10.0 max=40.0
  out "Expected position on spectrometer (pixels):":dbl
  out "Calibration Date: indicator:":u16(ring) items=["first calibration - 7/31", "7/31-current"]
  out "Harmonics Graph":cluster{"No prefix":dbl, i32}[](graph)
  out "Last image saved":string
  out "Bits/pixel":u16
  out "BufNr1":i16
  out "BufNr0":i16
  in  "ExposureTimeBase":u16(ring)=2 items=["nanoseconds", "microseconds", "milliseconds"]
  in  "Xmin":u16=760 min=1
  in  "Ymin":u16=410 min=1
  in  "Ymax":u16=1200 min=1
  in  "Xmax":u16=1560 min=1
  in  "Rate":i32(ring) items=["204000000", "0", "0", "0"]
  out "YResAct":u16
  out "XResAct":u16
  in  "Buffer0":bool
  in  "Buffer1":bool
  out "Horizontal resolution":u16
  out "Vertical resolution":u16
  in  "Exposure Time (secs)":sgl format="%.2f"
  out "Detector X Pixels":i32
  out "Detector Y Pixels":i32
  in  "Trigger":u32(ring) items=["Internal", "External"]
  out "Camera inputs":T6
  out "Camera outputs":T7
  out "Start Acquisition":u32
  out "Get Status":u32
  out "Status":u32
  out "Get Acquired Data":u32
  out "Shut Down":u32
  out "Image buffer":u64[](array[numeric])
  out "End of scan":bool
  # "Image Settings"
  # "Pump - probe scan Settings"
  # "Program Control"
  # "Analysis Settings"
  # "Saving Settings"
  # "Scan parameters"
  # "Y axis"
  # "VMI camera"
  # "XUV camera"
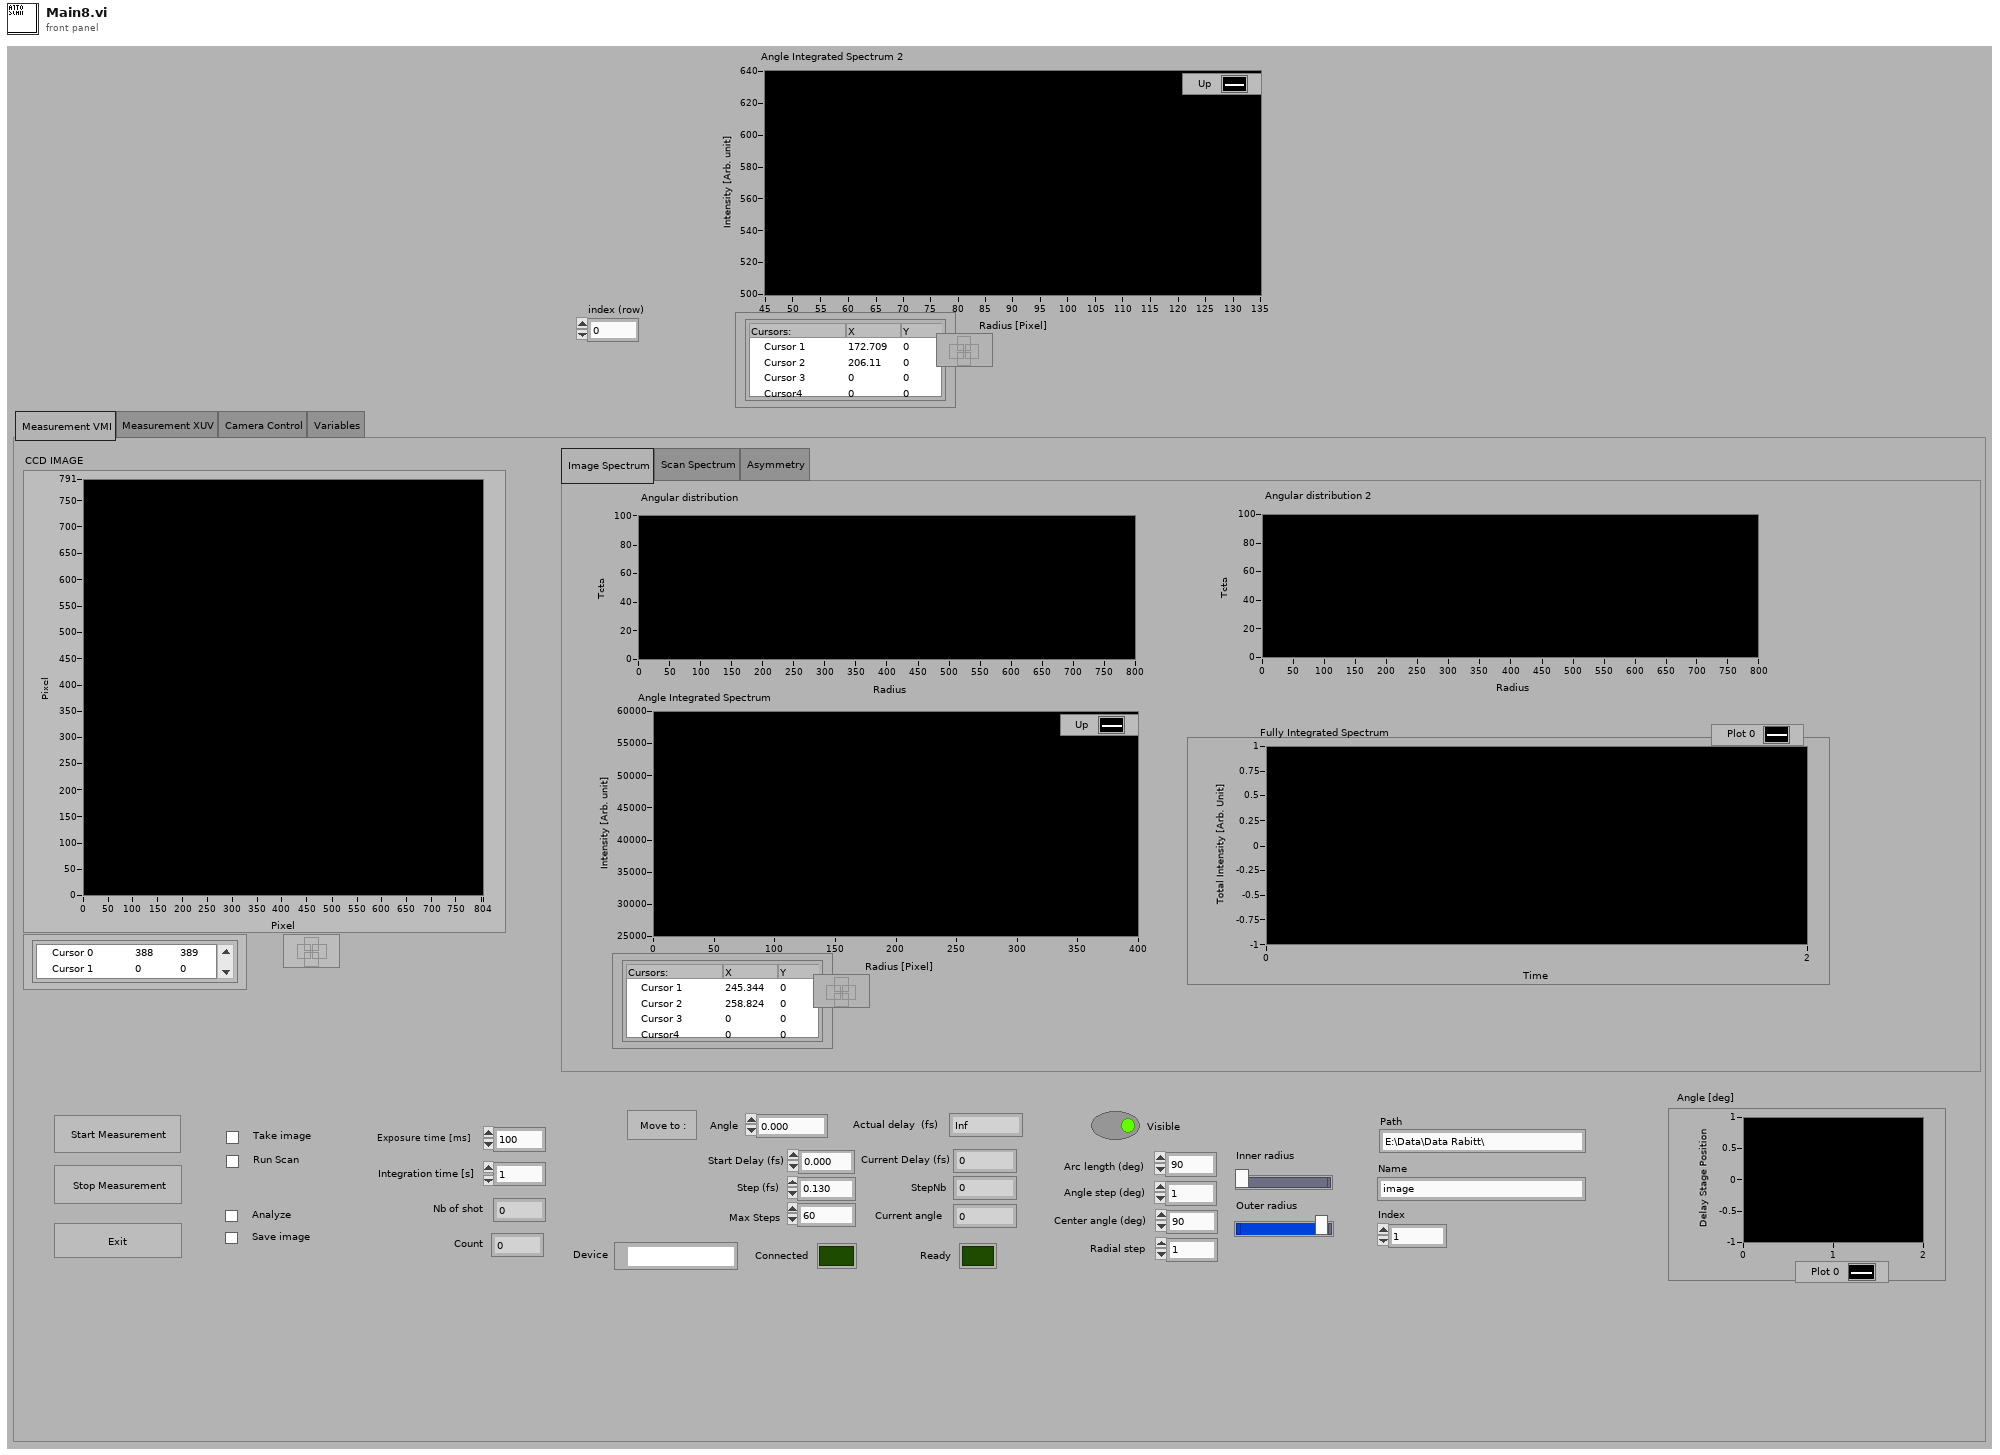
[diagram p1: front panel]
types:
  T1 = cluster{"Angle Sampling":dbl[], "Angle versus Radius Distribution":dbl[]}
  T2 = cluster{"Center angle (deg)":dbl, "Arc length (deg)":dbl, "Angle step (deg)":dbl, "Outer radius ":dbl, "Inner radius ":dbl, "Radius":dbl, "Radial step ":dbl}
  T3 = enum32{"Measurement VMI", "Measurement XUV", "Camera Control", "Variables"}
  T4 = enum32{"Image Spectrum", "Scan Spectrum", "Asymmetry"}
  T5 = cluster{"Radius Sampling":dbl[], "Angle Integrated Distribution":dbl[]}[]
  T6 = cluster{"Calculated Exposure Value":sgl, "Detector X Pixels":i32, "Detector Y Pixels":i32}
  T7 = cluster{"Initialize":u32, "Set Acquisition Mode":u32, "Set Readout Mode":u32, "Set Gate Mode":u32, "Get Detector":u32, "Set Image":u32, "Set Trigger Mode":u32, "Set Exposure Time":u32, "Check Timings":u32}
  T8 = cluster{"VISA resource name":refnum<visa-resource-name>, "Device name":string, "Controller address":i32, "error":errorcluster}
  T9 = typedef "LVRectTypeDef.ctl" = cluster{"Left":i16, "Top":i16, "Right":i16, "Bottom":i16}
  T10 = cluster{"to shutdown":bool, "to get acquired data":bool, "to start acquisition":bool, "DRV_SUCCESS":i32}
  T11 = cluster{"Size":u16, "SensorTypeDESC":u16, "SensorSubtypeDESC":u16, "MaxHorizontalResStdDESC":u16, "MaxVerticalResStdDESC":u16, "MaxHorizontalResExtDESC":u16, "MaxVerticalResExtDESC":u16, "DynResDESC":u16, "MaxBinHorzDESC":u16, "BinHorzStepDESC":bool, "MaxBinVertDESC":u16, "BinVertStepDESC":bool, "ROIHorzStepDESC":u16, "ROIVertStepDESC":u16, "NumADCDESC":u16, "IRDESC":bool, "MinDelayDESC":u32, "MaxDelayDESC":u32, "MinDelayStepDESC":u32, "MinExpoDESC":u32, "MaxExpoDESC":u32, "MinExpoStepDESC":u32, "MinDelayIRDESC":u32, "MaxDelayIRDESC":u32, "MinExpoIRDESC":u32, "MaxExpoIRDESC":u32, "TimeTableDESC":bool, "DoubleImageDESC":bool, "MinCoolSetDESC":i16, "MaxCoolSetDESC":i16, "MDefaultCoolSetDESC":i16, "PowerDownModeDESC":bool, "OffsetRegDESC":bool, "ColorPattern":cluster{"UpperLeftColor":u8, "UpperRightColor":u8, "LowerLeftColor":u8, "LowerRightColor":u8}, "PatternTypeDESC":bool, "PixelRates":u32[], "CoversionFactors":u16[], "Reserved":u32[], "GeneralCapabilities":u32, "GeneralCapabilities 2":u32, "Min Size Hor":u16, "Min Size Vert":u16, "Ext Synch Freq":u32[], "Cooling Setpoints":i16[], "Soft ROI Hor Step":u16, "Soft ROI Vert Step":u16}
  T12 = typedef "LVCursorListTypeDef.ctl" = cluster{"Name":string, "Color":u32, "Style":u8, "Point Style":u8, "Name Visible":bool, "Allow Drag":bool, "Cursor Mode":u32, "Plot":i32, "Index":i32, "Position":cluster{"X":dbl, "Y":dbl}, "X Scale":u32, "Y Scale":u32, "Watch Plots":i32[], "Watch All Plots":bool, "Plot Area":i32, "Label Offset":cluster{"X":dbl, "Y":dbl}}[]
  T13 = cluster{"Name":string, "Color":u32, "Style":u8, "Point Style":u8, "Name Visible":bool, "Allow Drag":bool, "Cursor Mode":u32, "Plot":i32, "Index":i32, "Position":cluster{"X":dbl, "Y":dbl}, "X Scale":u32, "Y Scale":u32, "Watch Plots":i32[], "Watch All Plots":bool, "Plot Area":i32, "Label Offset":cluster{"X":dbl, "Y":dbl}}
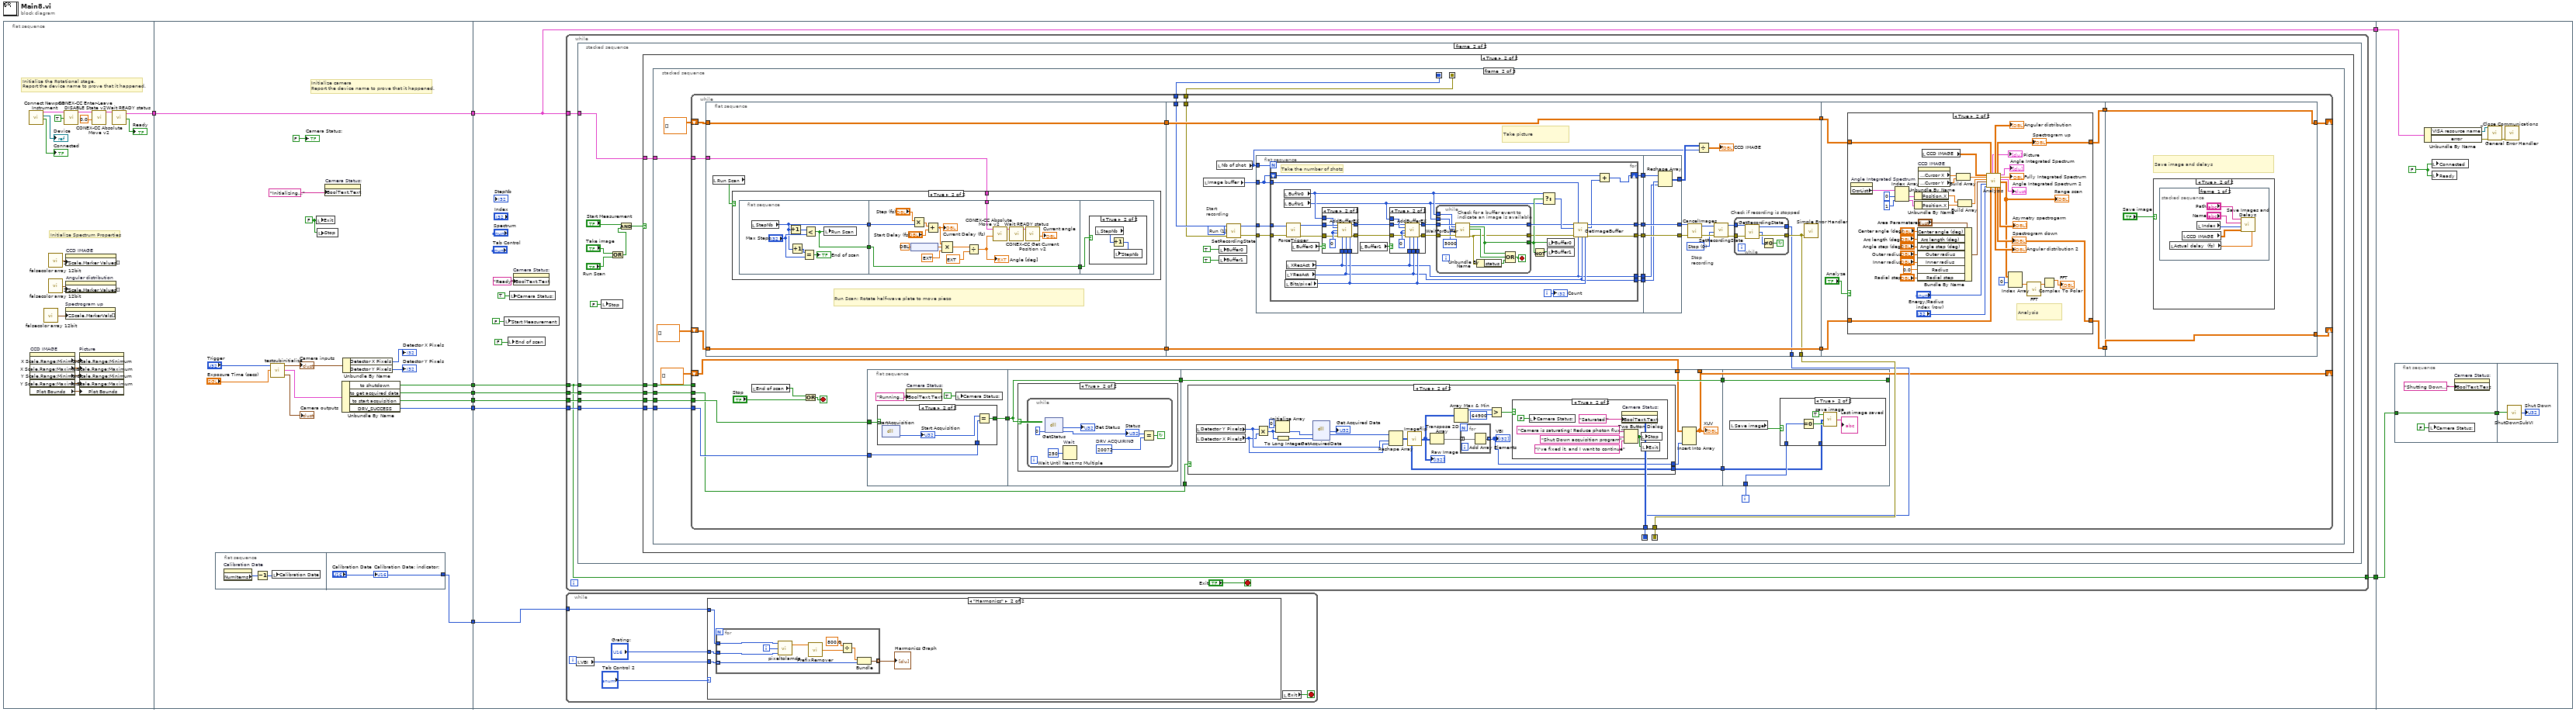
[diagram p0: block diagram]
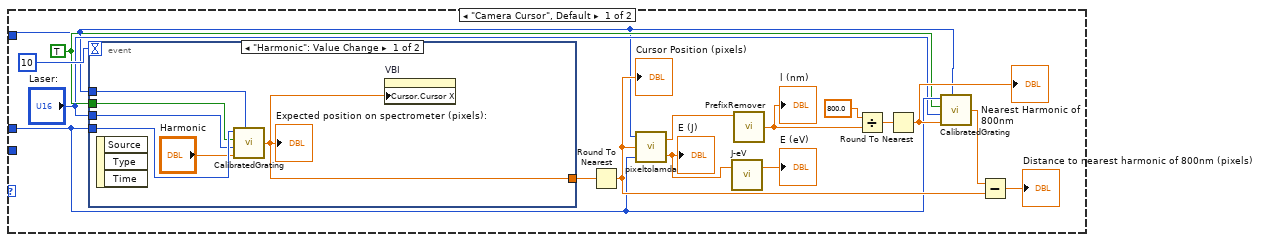
[diagram p2: hidden frame]
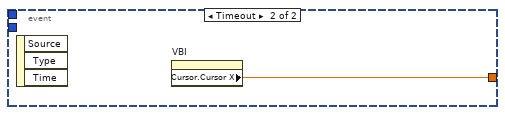
[diagram p3: hidden frame]
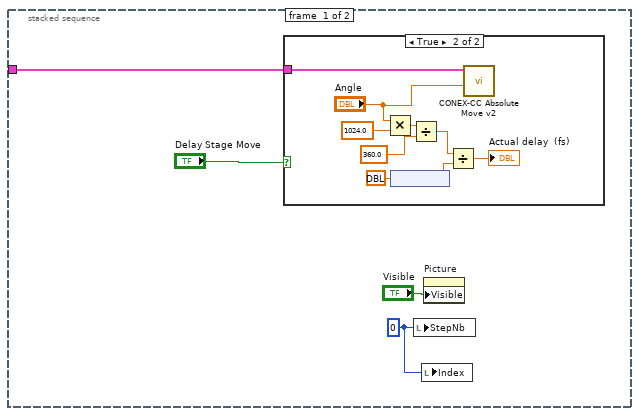
[diagram p4: hidden frame]
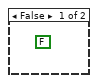
[diagram p6: hidden frame]
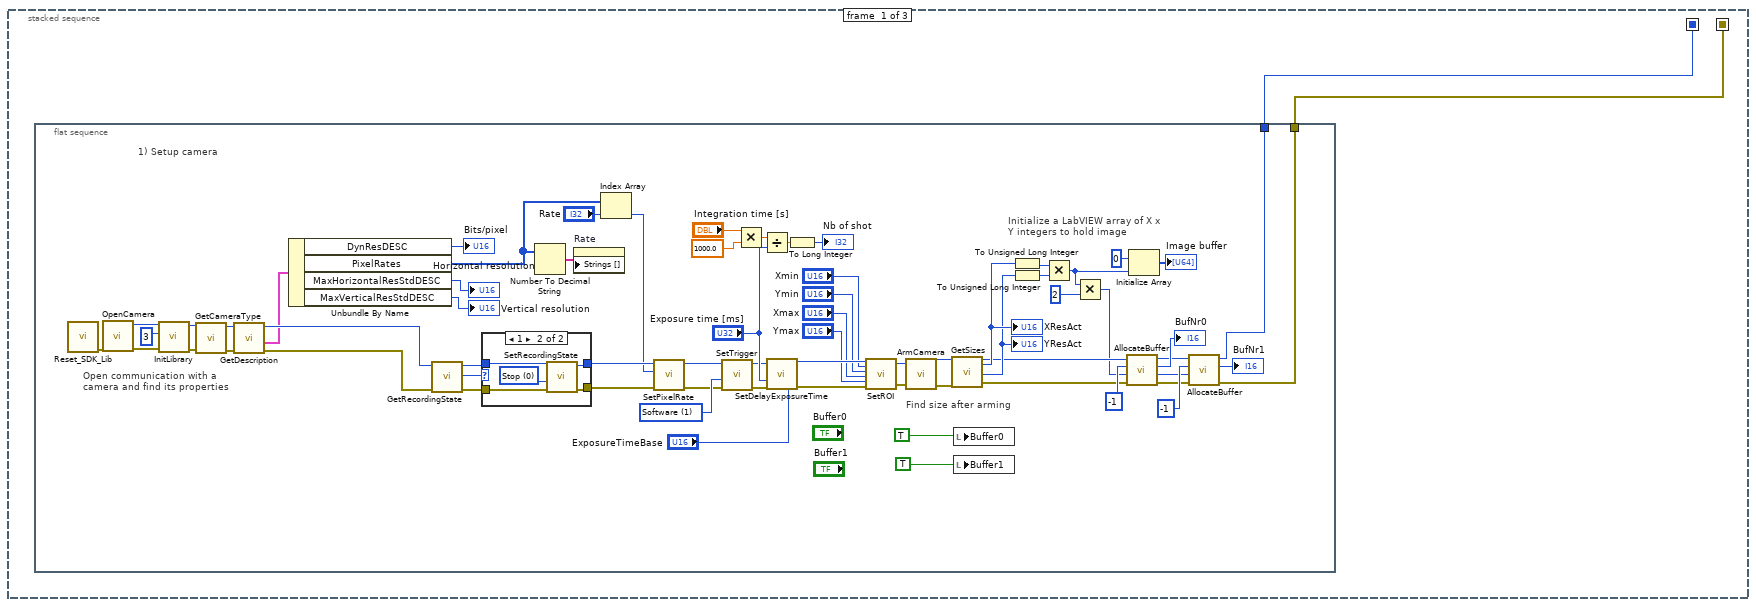
[diagram p7: hidden frame]
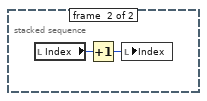
[diagram p20: hidden frame]
diagram:
  n1 = flat-sequence {
    tunnel: [w12] -> w8
    tunnel: w8 -> [w42]
    tunnel: [w42] -> w7
    tunnel: [w32] -> w6
    tunnel: [w31] -> w5
    tunnel: [w30] -> w4
    tunnel: [w29] -> w3
    tunnel: [w27] -> w1
    tunnel: w7 -> [w55]
    tunnel: [w55] -> w9
    tunnel: w6 -> [w54]
    tunnel: w5 -> [w53]
    tunnel: w4 -> [w52]
    tunnel: w3 -> [w51]
    tunnel: [w50] -> w2
    tunnel: w1 -> [w46]
    tunnel: w9 -> [w509]
    tunnel: w2 -> [w506]
    frame #0 {
      # "Initialize Spectrum Properties"
      # "Initialize the Rotational stage.\nReport the device name to prove that it happened."
      n2 = call <userlib>:"Connect Newport Instrument.vi"() -> ("Connected"=→"Connected":bool, "VISA resource name (duplicate)"=→"Device":refnum<visa-resource-name>, "Device Connection Cluster"=w16:T8)  [unwired: 7 in, 2 out]
      n3 = property on="CCD IMAGE" class="IntGraph (strict)"() -> ("X Scale.Range:Minimum"=w22:dbl, "X Scale.Range:Maximum"=w21:dbl, "Y Scale.Range:Minimum"=w20:dbl, "Y Scale.Range:Maximum"=w19:dbl, "Plot Bounds"=w23:T9)  [unwired: 2 in, 2 out]
      n4 = call "falsecolor array 12bit.vi"() -> ("Color Array"=w24:cluster{dbl, u32}[])  [unwired: 1 in]
      n5 = call "falsecolor array 12bit.vi"() -> ("Color Array"=w26:cluster{dbl, u32}[])  [unwired: 1 in]
      n6 = call "falsecolor array 12bit.vi"() -> ("Color Array"=w25:cluster{dbl, u32}[])  [unwired: 1 in]
      n7 = call <userlib>:"CONEX-CC Enter-Leave DISABLE State v2.vi"("Ready? (false=DISABLE true=READY)"=TRUE, "Connection Cluster in"=w16) -> ("Connection Cluster out"=w15:T8)  [unwired: 7 in]
      n8 = property on="Spectrogram up" class="IntGraph (strict)"("ZScale.MarkerVals[]"=w24) -> ()  [unwired: 2 in, 2 out]
      n9 = property on="CCD IMAGE" class="IntGraph (strict)"("Z Scale.Marker Values[]"=w26) -> ()  [unwired: 2 in, 2 out]
      n10 = property on="Angular distribution" class="IntGraph (strict)"("Z Scale.Marker Values[]"=w25) -> ()  [unwired: 2 in, 2 out]
      n11 = property on="Picture" class="XYGraph (strict)"("X Scale.Range:Minimum"=w22, "X Scale.Range:Maximum"=w21, "Y Scale.Range:Minimum"=w20, "Y Scale.Range:Maximum"=w19, "Plot Bounds"=w23) -> ()  [unwired: 2 in, 2 out]
      n12 = call <userlib>:"CONEX-CC Absolute Move v2.vi"("Target position"=0.0, "Connection Cluster in"=w15) -> ("Connection Cluster out"=w14:T8)  [unwired: 7 in]
      n13 = call <userlib>:"Wait READY status.vi"("Connection Cluster in"=w14) -> ("IsReady?"=→"Ready":bool, "Connection Cluster out"=w12:T8)  [unwired: 9 in]
    }
    frame #1 {
      w28 = FALSE ("Exit")
      # "Initialize camera\nReport the device name to prove that it happened."
      n14 = flat-sequence {
        tunnel: ["Calibration Date"] -> w27
        frame #0 {
          n15 = property on="Calibration Date" class="Ring (strict)"() -> ("NumItems"=w44:u32)  [unwired: 2 in, 2 out]
          n16 = Decrement(x=w44) -> (x-1=w43:u32)
          n17 = local write "Calibration Date"(w43) -> ()
        }
        frame #1 {
          "Calibration Date: indicator:" <- "Calibration Date"
        }
      }
      n18 = call "testsubinitialize.vi"("Exposure Time (secs)"="Exposure Time (secs)", "Trigger"="Trigger") -> ("Camera outputs"=→"Camera outputs":T7, "Camera status"=w35:T10, "Camera inputs"=w38:T6)  [unwired: 1 in]
      "Camera inputs" <- w38
      n19 = local write "Exit"(w28) -> ()
      n20 = local write "Stop"(w28) -> ()
      n21 = property on="Camera Status:" class="Bool (strict)"("BoolText.Text"="Initializing..." ("String")) -> ()  [unwired: 2 in, 2 out]
      n22 = Unbundle By Name(w35) -> ("to shutdown"=w32:bool, "to get acquired data"=w31:bool, "to start acquisition"=w30:bool, "DRV_SUCCESS"=w29:i32)
      n23 = Unbundle By Name(w38) -> ("Detector X Pixels"=→"Detector X Pixels":i32, "Detector Y Pixels"=→"Detector Y Pixels":i32)
      "Camera Status:" <- FALSE ("Camera Status:")
    }
    frame #2 {
      n24 = local write "Start Measurement"(FALSE) -> ()
      n25 = local write "End of scan"(FALSE) -> ()
      n26 = local write "Camera Status:"(TRUE ("Camera Status:")) -> ()
      n27 = property on="Camera Status:" class="Bool (strict)"("BoolText.Text"="Ready" ("Boolean Text.Text")) -> ()  [unwired: 2 in, 2 out]
      n28 = while {
        tunnel: w46 -> [w58]
        stop <- w59 stop-if-true
        n29 = local read "VBI"() -> (w57:i32[])
        n30 = case shown="\"Harmonics\"" "Tab Control 2" {
          tunnel: w57 -> [_ w88]
          tunnel: "Grating:" -> [w65 w87]
          tunnel: w58 -> [w62 w85]
          frame "Camera Cursor", Default {
            w64 = TRUE
            n31 = event shown="[0] \"Harmonic\": Value Change" {
              selector: _ -> [_ _]
              dyn-events: _ -> [_ _]
              timeout: 10 -> [_ _]
              tunnel: [w78 w84] -> w66
              tunnel: w65 -> [w83 _]
              tunnel: w64 -> [w82 _]
              tunnel: "Laser:" -> [w81 _]
              tunnel: w62 -> [w80 _]
              event "Harmonic": Value Change {
                n32 = event-data() -> ()  [unwired: 1 in, 3 out]
                n33 = call "CalibratedGrating.vi"("Grating:"=w83, "Subvi?"=w82, "Laser:"=w81, "Harmonic"="Harmonic", "Caibration Date"=w80) -> ("Position on spectrometer (pixels):"=w78:dbl)
                "Expected position on spectrometer (pixels):" <- w78
                n34 = property on="VBI" class="WFGraph (strict)"("Cursor.Cursor X"=w78) -> ()  [unwired: 2 in, 2 out]
              }
              event Timeout {
                n35 = event-data() -> ()  [unwired: 1 in, 3 out]
                n36 = property on="VBI" class="WFGraph (strict)"() -> ("Cursor.Cursor X"=w84:dbl)  [unwired: 2 in, 2 out]
              }
            }
            n37 = Round To Nearest(number=w66) -> (nearest integer value=w71:dbl)
            "Cursor Position (pixels)" <- w71
            n38 = call "pixeltolamda.vi"("Grating:"=w65, "Pixel Postion"=w71, "Caibration Date"=w62) -> ("E (J)"=w73:dbl, "lamda (m)"=w77:dbl)
            "E (J)" <- w73
            n39 = call "J-eV.vi"("J"=w73) -> ("eV"=→"E (eV)":dbl)  [unwired: 1 in, 1 out]
            n40 = call "PrefixRemover.vi"("Nano"=w77) -> ("No prefix"=w74:dbl)  [unwired: 3 in]
            "l (nm)" <- w74
            n41 = Divide(x=800.0, y=w74) -> (x/y=w76:dbl)
            n42 = Round To Nearest(number=w76) -> (nearest integer value=w70:dbl)
            "Nearest Harmonic of 800nm" <- w70
            n43 = call "CalibratedGrating.vi"("Grating:"=w65, "Subvi?"=w64, "Laser:"="Laser:", "Harmonic"=w70, "Caibration Date"=w62) -> ("Position on spectrometer (pixels):"=w69:dbl)
            n44 = Subtract(x=w69, y=w71) -> (x-y=→"Distance to nearest harmonic of 800nm (pixels)":dbl)
          }
          frame "Harmonics" {
            n45 = for {
              tunnel: w88 -> [w94] mode=indexing
              tunnel: w87 -> [w96]
              tunnel: [w93] -> w86 mode=indexing
              tunnel: w85 -> [w89]
              i -> [w95]
              n46 = call "pixeltolamda.vi"("Grating:"=w96, "Pixel Postion"=w95, "Caibration Date"=w89) -> ("lamda (m)"=w97:dbl)  [unwired: 1 out]
              n47 = call "PrefixRemover.vi"("Nano"=w97) -> ("No prefix"=w91:dbl)  [unwired: 3 in]
              n48 = Divide(x=800.0, y=w91) -> (x/y=w90:dbl)
              n49 = Bundle(w90, w94) -> (w93:cluster{dbl, i32})  [unwired: 1 in]
            }
            "Harmonics Graph" <- w86
          }
        }
        n50 = local read "Exit"() -> (w59:bool)
      }
      n51 = while {
        tunnel: w55 -> [w102]
        tunnel: w54 -> [w98]
        tunnel: w53 -> [w101]
        tunnel: w52 -> [w100]
        tunnel: w51 -> [w99]
        tunnel: [w98] -> w50
        stop <- "Exit" stop-if-true
        n52 = stacked-sequence {
          tunnel: w102 -> [w105 w122]
          tunnel: w98 -> [_ w121]
          tunnel: w101 -> [_ w120]
          tunnel: w100 -> [_ w119]
          tunnel: w99 -> [_ w118]
          frame #0 {
            w104 = 0 ("Done Step")
            n53 = case shown="True" "Delay Stage Move" {
              tunnel: w105 -> [_ w110]
              frame False {
              }
              frame True {
                n54 = Multiply(x="Angle", y=1024.0) -> (x*y=w115:dbl)
                n55 = node(ext[unit] 299792458.0) -> (w111:ext)
                n56 = Divide(x=w115, y=360.0) -> (x/y=w113:dbl)
                n57 = Divide(x=w113, y=w111) -> (x/y=→"Actual delay  (fs)":ext)
                n58 = call <userlib>:"CONEX-CC Absolute Move v2.vi"("Target position"="Angle", "Connection Cluster in"=w110) -> ()  [unwired: 7 in, 1 out]
              }
            }
            n59 = local write "StepNb"(w104) -> ()
            n60 = local write "Index"(w104) -> ()
            n61 = property on="Picture" class="XYGraph (strict)"("Visible"="Visible") -> ()  [unwired: 2 in, 2 out]
          }
          frame #1 {
            n62 = local write "Stop"(FALSE ("Stop")) -> ()
            n63 = Or(x="Take image", y="Run Scan") -> (x .or. y?=w123:bool)
            n64 = And(x="Start Measurement", y=w123) -> (x .and. y?=w125:bool)
            n65 = case shown="True" w125 {
              tunnel: w122 -> [_ w132]
              tunnel: w121 -> [_ w131]
              tunnel: w120 -> [_ w130]
              tunnel: w119 -> [_ w129]
              tunnel: w118 -> [_ w128]
              frame False {
                (unwired) FALSE
              }
              frame True {
                n66 = stacked-sequence {
                  seq-local: [_ w217 _] -> [_ _ w501]
                  seq-local: [_ w216 _] -> [_ _ w500]
                  seq-local: [w133 _ _] -> [_ w214 _]
                  seq-local: [w134 _ _] -> [_ w215 _]
                  tunnel: w132 -> [_ w213 _]
                  tunnel: w131 -> [_ w212 _]
                  tunnel: w130 -> [_ w211 _]
                  tunnel: w129 -> [_ w210 _]
                  tunnel: w128 -> [_ w209 _]
                  frame #0 {
                    n67 = flat-sequence {
                      tunnel: [w136] -> w133
                      tunnel: [w135] -> w134
                      frame #0 {
                        w172 = u16 1 items=["Auto", "Software", "External sequence start ", "External exposure control"] ("TriggerMode")
                        # "Find size after arming"
                        # "1) Setup camera"
                        # "Initialize a LabVIEW array of X x Y integers to hold image"
                        # "Open communication with a camera and find its properties"
                        n68 = call "Reset_SDK_Lib.vi"() -> ("ErrorOut"=w157:errorcluster)  [unwired: 11 in]
                        n69 = call "OpenCamera.vi"("ErrorIn"=w157) -> ("ErrorOut"=w148:errorcluster, "Handle out"=w147:u64)  [unwired: 3 in, 2 out]
                        n70 = call "InitLibrary.vi"("error in (no error)"=w148, "InterfaceType"=u32 3, "ph"=w147) -> ("error out"=w149:errorcluster, "hout"=w150:u64)  [unwired: 7 in]
                        n71 = call "GetCameraType.vi"("ph"=w150, "error in (no error)"=w149) -> ("hout"=w141:u64, "error out"=w142:errorcluster)  [unwired: 1 in, 2 out]
                        n72 = call "GetDescription.vi"("ErrorIn"=w142, "ph"=w141) -> ("ErrorOut"=w152:errorcluster, "Description"=w140:T11, "hout"=w153:u64)  [unwired: 2 in, 1 out]
                        n73 = Unbundle By Name(w140) -> ("DynResDESC"=→"Bits/pixel":u16, "PixelRates"=w171:u32[], "MaxHorizontalResStdDESC"=→"Horizontal resolution":u16, "MaxVerticalResStdDESC"=→"Vertical resolution":u16)
                        n74 = call "GetRecordingState.vi"("ErrorIn"=w152, "ph"=w153) -> ("ErrorOut"=w155:errorcluster, "Error"=w156:i32, "hout"=w154:u64)  [unwired: 2 in, 1 out]
                        n75 = case shown="1" w156 {
                          tunnel: w154 -> [w202 w206]
                          tunnel: w155 -> [w201 w205]
                          tunnel: [w202 w204] -> w189
                          tunnel: [w201 w203] -> w190
                          frame 0, Default {
                          }
                          frame 1 {
                            w207 = u16 0 items=["Stop", "Run"] ("RecordingState")
                            n76 = call "SetRecordingState.vi"("ErrorIn"=w205, "RecordingState"=w207, "ph"=w206) -> ("ErrorOut"=w203:errorcluster, "hout"=w204:u64)  [unwired: 2 in, 1 out]
                          }
                        }
                        n77 = Number To Decimal String(number=w171) -> (decimal integer string=w146:string[])  [unwired: 1 in]
                        n78 = property on="Rate" class="Ring (strict)"("Strings []"=w146) -> ()  [unwired: 2 in, 2 out]
                        n79 = Index Array(array=w171, index="Rate") -> (element=w170:u32)
                        n80 = call "SetPixelRate.vi"("error in (no error)"=w190, "PixelRate"=w170, "ph"=w189) -> ("error out"=w161:errorcluster, "hout"=w162:u64)  [unwired: 2 in, 1 out]
                        n81 = call "SetTrigger.vi"("error in (no error)"=w161, "TriggerMode"=w172, "ph"=w162) -> ("error out"=w168:errorcluster, "hout"=w169:u64)  [unwired: 2 in, 1 out]
                        n82 = Multiply(x="Integration time [s]", y=1000.0) -> (x*y=w196:dbl)
                        n83 = Divide(x=w196, y="Exposure time [ms]") -> (x/y=w198:dbl)
                        n84 = call "SetDelayExposureTime.vi"("ph"=w169, "Exposure"="Exposure time [ms]", "error in (no error)"=w168, "ExposureTimeBase"="ExposureTimeBase") -> ("hout"=w166:u64, "error out"=w165:errorcluster)  [unwired: 9 in, 1 out]
                        n85 = To Long Integer(number=w198) -> (32bit integer=→"Nb of shot":i32)
                        n86 = call "SetROI.vi"("ph"=w166, "ROIX0"="Xmin", "ROIY0"="Ymin", "ROIX1"="Xmax", "ROIY1"="Ymax", "error in (no error)"=w165) -> ("hout"=w183:u64, "error out"=w184:errorcluster)  [unwired: 12 in]
                        n87 = call "ArmCamera.vi"("error in (no error)"=w184, "ph"=w183) -> ("error out"=w181:errorcluster, "hout"=w182:u64)  [unwired: 1 in, 1 out]
                        n88 = call "GetSizes.vi"("ph"=w182, "ErrorIn"=w181) -> ("hout"=w179:u64, "XResAct"=w200:u16, "YResAct"=w199:u16, "ErrorOut"=w180:errorcluster)  [unwired: 11 in, 3 out]
                        "YResAct" <- w199
                        "XResAct" <- w200
                        n89 = local write "Buffer0"(TRUE) -> ()
                        n90 = local write "Buffer1"(TRUE) -> ()
                        n91 = To Unsigned Long Integer(number=w200) -> (unsigned 32bit integer=w176:u32)
                        n92 = To Unsigned Long Integer(number=w199) -> (unsigned 32bit integer=w177:u32)
                        n93 = Multiply(x=w176, y=w177) -> (x*y=w186:u32)
                        n94 = Multiply(x=w186, y=u32 2) -> (x*y=w173:u32)
                        n95 = call "AllocateBuffer.vi"("error in (no error)"=w180, "Size"=w173, "BufNr"=i16 -1, "ph"=w179) -> ("error out"=w175:errorcluster, "BufNrOut"=→"BufNr0":i16, "hout"=w174:u64)  [unwired: 2 in, 3 out]
                        n96 = Initialize Array(u16 0 ("Element Data"), w186) -> (→"Image buffer":u16[])
                        n97 = call "AllocateBuffer.vi"("error in (no error)"=w175, "Size"=w173, "BufNr"=i16 -1, "ph"=w174) -> ("error out"=w135:errorcluster, "BufNrOut"=→"BufNr1":i16, "hout"=w136:u64)  [unwired: 2 in, 3 out]
                      }
                    }
                  }
                  frame #1 {
                    n98 = while {
                      shift-right: [w246] -> _
                      shift-left: dbl[][] [] -> [w247]
                      shift-right: [w244] -> _
                      shift-left: dbl[][] [] -> [w245]
                      tunnel: [w236] -> w217
                      tunnel: [w235] -> w216
                      tunnel: w214 -> [w234]
                      tunnel: w215 -> [w233]
                      tunnel: w213 -> [w232]
                      tunnel: w212 -> [_]
                      tunnel: w211 -> [w227]
                      tunnel: w210 -> [w228]
                      tunnel: w209 -> [w229]
                      shift-right: [w222] -> _
                      shift-left: dbl[][] [] -> [w220]
                      i -> [w221]
                      stop <- w243 stop-if-true
                      n99 = flat-sequence {
                        tunnel: w247 -> [w304]
                        tunnel: [w304] -> w240
                        tunnel: w245 -> [w303]
                        tunnel: [w303] -> w239
                        tunnel: w232 -> [w302]
                        tunnel: w240 -> [w344]
                        tunnel: [w344] -> w238
                        tunnel: w239 -> [w343]
                        tunnel: [w343] -> w237
                        tunnel: w234 -> [w342]
                        tunnel: w233 -> [w341]
                        tunnel: [w340] -> w236
                        tunnel: [w339] -> w235
                        tunnel: w238 -> [w447]
                        tunnel: [w445] -> w226
                        tunnel: w237 -> [w444]
                        tunnel: [w443] -> w225
                        tunnel: [w490] -> w246
                        tunnel: w226 -> [w490]
                        tunnel: [w489] -> w244
                        tunnel: w225 -> [w489]
                        frame #0 {
                          # "Run Scan: Rotate half-wave plate to move piezo"
                          n100 = local read "Run Scan"() -> (w305:bool)
                          n101 = case shown="True" w305 {
                            tunnel: w302 -> [_ w306]
                            frame False {
                            }
                            frame True {
                              n102 = flat-sequence {
                                tunnel: [w314] -> w309
                                tunnel: [w311] -> w308
                                tunnel: w309 -> [w329]
                                tunnel: w308 -> [w330]
                                tunnel: [w329] -> w307
                                tunnel: w306 -> [w318]
                                tunnel: w307 -> [w332]
                                frame #0 {
                                n103 = local read "StepNb"() -> (w311:i32)
                                n104 = Increment(x=w311) -> (x+1=w310:i32)
                                n105 = Increment(x=w311) -> (x+1=w315:i32)
                                n106 = Equal?(x=w315, y="Max Steps") -> (x = y?=→"End of scan":bool)
                                n107 = Less?(x=w310, y="Max Steps") -> (x < y?=w314:bool)
                                n108 = local write "Run Scan"(w314) -> ()
                                }
                                frame #1 {
                                n109 = node(ext[unit] 299792458.0) -> (w325:ext)
                                n110 = Multiply(x="Step (fs)", y=w330) -> (x*y=w328:dbl)
                                n111 = Add(x=w328, y="Start Delay (fs)") -> (x+y=w323:dbl)
                                "Current Delay (fs)" <- w323
                                n112 = Compound Arithmetic op=MULTIPLY(w323, w325, ext 360.0 ("y")) -> (w317:ext)
                                n113 = Divide(x=w317, y=ext 2128.0) -> (x/y=w319:ext)
                                "Angle [deg]" <- w319
                                n114 = call <userlib>:"CONEX-CC Absolute Move v2.vi"("Target position"=w319, "Connection Cluster in"=w318) -> ("Connection Cluster out"=w322:T8)  [unwired: 7 in]
                                n115 = call <userlib>:"Wait READY status.vi"("Connection Cluster in"=w322) -> ("Connection Cluster out"=w321:T8)  [unwired: 9 in, 1 out]
                                n116 = call <userlib>:"CONEX-CC Get Current Position v2.vi"("Connection Cluster in"=w321) -> ("Current position"=→"Current angle":dbl)  [unwired: 8 in, 2 out]
                                }
                                frame #2 {
                                n117 = case shown="True" w332 {
                                frame False {
                                }
                                frame True {
                                n118 = local read "StepNb"() -> (w334:i32)
                                n119 = Increment(x=w334) -> (x+1=w333:i32)
                                n120 = local write "StepNb"(w333) -> ()
                                }
                                }
                                }
                              }
                            }
                          }
                        }
                        frame #1 {
                          w348 = u16 1 items=["Stop", "Run"] ("RecordingState")
                          w345 = u16 0 items=["Stop", "Run"] ("RecordingState")
                          # "Check if recording is stopped"
                          # "Start recording"
                          # "Stop recording"
                          # "Take picture"
                          n121 = local read "Image buffer"() -> (w338:u64[])
                          n122 = local read "Nb of shot"() -> (w336:i32)
                          n123 = local write "Buffer0"(TRUE) -> ()
                          n124 = local write "Buffer1"(TRUE) -> ()
                          n125 = call "SetRecordingState.vi"("ErrorIn"=w341, "RecordingState"=w348, "ph"=w342) -> ("ErrorOut"=w356:errorcluster, "hout"=w355:u64)  [unwired: 2 in, 1 out]
                          n126 = flat-sequence {
                            tunnel: [w370] -> w361
                            tunnel: [w369] -> w360
                            tunnel: [w366] -> w359
                            tunnel: [w365] -> w358
                            tunnel: [w364] -> w357
                            tunnel: w355 -> [w368]
                            tunnel: w356 -> [w367]
                            tunnel: w338 -> [w362]
                            tunnel: w336 -> [w363]
                            tunnel: w361 -> [w436]
                            tunnel: w360 -> [w435]
                            tunnel: w359 -> [w433]
                            tunnel: w358 -> [w432]
                            tunnel: w357 -> [w434]
                            tunnel: [w436] -> w354
                            tunnel: [w435] -> w353
                            tunnel: [w431] -> w337
                            frame #0 {
                              n127 = for {
                                N: w363 -> [_]
                                tunnel: [w376] -> w366
                                tunnel: [w375] -> w365
                                tunnel: w368 -> [w383]
                                tunnel: [w396] -> w369
                                tunnel: w367 -> [w382]
                                tunnel: [w397] -> w370
                                tunnel: w362 -> [w395]
                                shift-right: [w371] -> w364
                                shift-left: w362 -> [w373]
                                i -> [w372]
                                # "Take the number of shots"
                                n128 = local read "BufNr0"() -> (w378:i16)
                                n129 = local read "BufNr1"() -> (w377:i16)
                                n130 = local read "Bits/pixel"() -> (w379:u16)
                                n131 = local read "YResAct"() -> (w376:u16)
                                n132 = call "ForceTrigger.vi"("ph"=w383, "error in (no error)"=w382) -> ("hout"=w380:u64, "error out"=w381:errorcluster)  [unwired: 1 in, 2 out]
                                n133 = local read "XResAct"() -> (w375:u16)
                                n134 = local read "Buffer0"() -> (w392:bool)
                                n135 = case shown="True" w392 {
                                tunnel: [w399 w408] -> w393
                                tunnel: [w398 w407] -> w394
                                tunnel: w378 -> [_ w400]
                                tunnel: w380 -> [w398 w406]
                                tunnel: w379 -> [_ w404]
                                tunnel: w375 -> [_ w403]
                                tunnel: w376 -> [_ w402]
                                tunnel: w381 -> [w399 w401]
                                frame False {
                                }
                                frame True {
                                w405 = i16 0
                                n136 = call "AddBufferEX.vi"("ph"=w406, "BuffNr"=w400, "1stImage"=w405, "LastImage"=w405, "error in (no error)"=w401, "XRes"=w403, "YRes"=w402, "BitPerPixel"=w404) -> ("hout"=w407:u64, "error out"=w408:errorcluster)  [unwired: 5 in, 1 out]
                                }
                                }
                                n137 = local read "Buffer1"() -> (w391:bool)
                                n138 = case shown="True" w391 {
                                tunnel: [w409 w419] -> w387
                                tunnel: [w410 w418] -> w388
                                tunnel: w377 -> [_ w417]
                                tunnel: w394 -> [w410 w416]
                                tunnel: w379 -> [_ w414]
                                tunnel: w375 -> [_ w413]
                                tunnel: w376 -> [_ w412]
                                tunnel: w393 -> [w409 w411]
                                frame False {
                                }
                                frame True {
                                w415 = i16 0
                                n139 = call "AddBufferEX.vi"("ph"=w416, "BuffNr"=w417, "1stImage"=w415, "LastImage"=w415, "error in (no error)"=w411, "XRes"=w413, "YRes"=w412, "BitPerPixel"=w414) -> ("hout"=w418:u64, "error out"=w419:errorcluster)  [unwired: 5 in, 1 out]
                                }
                                }
                                n140 = while {
                                tunnel: w378 -> [w427]
                                tunnel: w377 -> [w426]
                                tunnel: w388 -> [w429]
                                tunnel: w387 -> [w428]
                                tunnel: [w425] -> w386
                                tunnel: [w421] -> w384
                                tunnel: [w424] -> w385
                                stop <- w430 stop-if-true
                                # "Check for a buffer event to indicate an image is available"
                                n141 = call "WaitForBuffer.vi"("ph"=w429, "sBufNr"=w427, "sBufNr 2"=w426, "timeout"=5000, "error in (no error)"=w428) -> ("hout"=w425:u64, "Buffer_Ready"=w424:bool, "Buffer_Ready 2"=w423:bool, "error out"=w421:errorcluster)  [unwired: 10 in, 1 out]
                                n142 = Unbundle By Name(w421) -> ("status"=w420:bool)
                                n143 = Compound Arithmetic op=OR(w424, w423, w420) -> (w430:bool)
                                }
                                n144 = Not(x=w385) -> (.not. x?=w389:bool)
                                n145 = Select(t=w378, s=w385, f=w377) -> (s? t:f=w390:i16)
                                n146 = local write "Buffer0"(w385) -> ()
                                n147 = local write "Buffer1"(w389) -> ()
                                n148 = call "GetImageBuffer.vi"("ph"=w386, "BuffIn"=w395, "BuffNr"=w390, "error in (no error)"=w384, "xRes"=w375, "yRes"=w376, "Bitresolution"=w379) -> ("hout"=w396:u64, "BuffOut"=w374:u16[], "error out"=w397:errorcluster)  [unwired: 5 in, 1 out]
                                n149 = Add(x=w373, y=w374) -> (x+y=w371:u64[])
                                "Count" <- w372
                              }
                            }
                            frame #1 {
                              n150 = Reshape Array(w434, w433, w432) -> (w431:u64[][])
                            }
                          }
                          n151 = call "CancelImages.vi"("error in (no error)"=w354, "ph"=w353) -> ("error out"=w351:errorcluster, "hout"=w352:u64)  [unwired: 1 in, 1 out]
                          n152 = Divide(x=w337, y=w336) -> (x/y=→"CCD IMAGE":dbl[][])
                          n153 = call "SetRecordingState.vi"("ErrorIn"=w351, "RecordingState"=w345, "ph"=w352) -> ("ErrorOut"=w347:errorcluster, "hout"=w346:u64)  [unwired: 2 in, 1 out]
                          n154 = while {
                            tunnel: [w440] -> w340
                            tunnel: w347 -> [w441]
                            tunnel: w346 -> [w442]
                            tunnel: [w437] -> w339
                            stop <- w438 continue-if-true
                            n155 = call "GetRecordingState.vi"("ErrorIn"=w441, "ph"=w442) -> ("ErrorOut"=w440:errorcluster, "RecordingState"=w439:u16, "hout"=w437:u64)  [unwired: 2 in, 1 out]
                            n156 = Not Equal To 0?(x=w439) -> (x != 0?=w438:bool)
                          }
                          n157 = call <vilib>:"Simple Error Handler.vi"("error in (no error)"=w340) -> ()  [unwired: 4 in, 5 out]
                        }
                        frame #2 {
                          n158 = case shown="True" "Analyze" {
                            tunnel: w447 -> [w449 w476]
                            tunnel: [w449 w463] -> w445
                            tunnel: w444 -> [w448 w472]
                            tunnel: [w448 w462] -> w443
                            frame False {
                            }
                            frame True {
                              # "Analysis"
                              n159 = property on="Angle Integrated Spectrum" class="XYGraph (strict)"() -> ("CrsrList"=w479:T12)  [unwired: 2 in, 2 out]
                              n160 = Index Array(array=w479, index #1=0, index #2=1) -> (element #1=w461:T13, element #2=w460:T13)
                              n161 = Unbundle By Name(w461) -> ("Position.X"=w459:dbl)
                              n162 = Unbundle By Name(w460) -> ("Position.X"=w458:dbl)
                              n163 = Bundle By Name(cluster="Area Parameteres", "Center angle (deg)"="Center angle (deg)", "Arc length (deg)"="Arc length (deg)", "Angle step (deg)"="Angle step (deg)", "Outer radius"="Outer radius", "Inner radius"="Inner radius", "Radius"=0.0 ("Arc length (deg)"), "Radial step"="Radial step") -> (w473:T2)
                              n164 = property on="CCD IMAGE" class="IntGraph (strict)"() -> ("Cursor.Cursor Position:Cursor X"=w475:dbl, "Cursor.Cursor Position:Cursor Y"=w474:dbl)  [unwired: 2 in, 2 out]
                              n165 = local read "CCD IMAGE"() -> (w477:dbl[][])
                              n166 = Build Array(w475, w474) -> (w457:dbl[])
                              n167 = Build Array(w459, w458) -> (w456:dbl[])
                              n168 = call "Analysis.vi"("CCD image"=w477, "CCD image Cursor position"=w457, "Angle integrated Cursor position"=w456, "Area Parameters"=w473, "Energy/Radius"="Energy/Radius", "index (row)"="index (row)", "Spec Up"=w476, "Spec Down"=w472) -> ("Picture"=→"Picture":cluster{dbl[], dbl[]}[], "Angular distribution"=→"Angular distribution":dbl[][], "Angular distribution 2"=→"Angular distribution 2":dbl[][], "Spectrogram Up"=w463:dbl[][], "Spectrogram Down"=w462:dbl[][], "Angle Integrated Spectrum"=→"Angle Integrated Spectrum":T5, "Fully Integrated Spectrum"=→"Fully Integrated Spectrum":dbl, "Angle Integrated Spectrum 2"=→"Angle Integrated Spectrum 2":T1, "Range scan"=w454:dbl[][], "Asymetry Spectrogram"=→"Asymetry spectrogarm":dbl[][])  [unwired: 1 in, 1 out]
                              "Range scan" <- w454
                              "Spectrogram up" <- w463
                              "Spectrogram down" <- w462
                              n169 = Index Array(array=w454, index (row)=0) -> (element=w452:dbl[])  [unwired: 1 in]
                              n170 = call-poly <vilib>:"FFT.vi"("X"=w452) -> ("FFT {X}"=w451:cdb[])  [unwired: 9 in, 1 out]
                              n171 = Complex To Polar(r * e^(i*theta)=w451) -> (r=→"FFT":dbl[])  [unwired: 1 out]
                            }
                          }
                        }
                        frame #3 {
                          # "Save image and delays"
                          n172 = case shown="True" "Save image" {
                            frame False {
                            }
                            frame True {
                              n173 = stacked-sequence {
                                frame #0 {
                                n174 = local read "Actual delay  (fs)"() -> (w496:dbl)
                                n175 = local read "CCD IMAGE"() -> (w495:dbl[][])
                                n176 = local read "Index"() -> (w494:i32)
                                n177 = call "Save Images and Delays.vi"("Delay [fs]"=w496, "Array"=w495, "Index"=w494, "Name"="Name", "Path"="Path") -> ()
                                }
                                frame #1 {
                                n178 = local read "Index"() -> (w498:i32)
                                n179 = Increment(x=w498) -> (x+1=w497:i32)
                                n180 = local write "Index"(w497) -> ()
                                }
                              }
                            }
                          }
                        }
                      }
                      n181 = local read "End of scan"() -> (w241:bool)
                      n182 = Or(x=w241, y="Stop") -> (x .or. y?=w243:bool)
                      n183 = flat-sequence {
                        tunnel: [w252] -> w231
                        tunnel: w229 -> [w249]
                        tunnel: w228 -> [w248]
                        tunnel: w231 -> [w257]
                        tunnel: [w257] -> w230
                        tunnel: w230 -> [w269]
                        tunnel: w227 -> [w268]
                        tunnel: [w269] -> w224
                        tunnel: [w267] -> w223
                        tunnel: w220 -> [w266]
                        tunnel: [w264] -> w222
                        tunnel: [w296] -> _
                        tunnel: w224 -> [w296]
                        tunnel: w223 -> [w294]
                        tunnel: w221 -> [w295]
                        frame #0 {
                          n184 = case shown="True" w248 {
                            tunnel: [FALSE w256] -> w252
                            tunnel: w249 -> [_ w254]
                            frame False {
                            }
                            frame True {
                              n185 = dll-call lib="atmcd32d.dll" fn="StartAcquisition" label="Call Library Function start acquisition"() -> (w255:u32)  [unwired: 3 in, 2 out]
                              "Start Acquisition" <- w255
                              n186 = Equal?(x=w255, y=w254) -> (x = y?=w256:bool)
                            }
                          }
                          n187 = property on="Camera Status:" class="Bool (strict)"("BoolText.Text"="Running..." ("Boolean Text.Text")) -> ()  [unwired: 2 in, 2 out]
                          n188 = local write "Camera Status:"(TRUE ("Camera Status:")) -> ()
                        }
                        frame #1 {
                          n189 = case shown="True" w257 {
                            frame False {
                            }
                            frame True {
                              n190 = while {
                                stop <- w261 continue-if-true
                                w260 = u16 20072  # DRV ACQUIRING
                                n191 = dll-call lib="atmcd32d.dll" fn="GetStatus" label="Call Library Function GetAcquisitionStatus"(u16 0) -> (→"Get Status":u32, w259:u32)  [unwired: 3 in, 2 out]
                                "Status" <- w259
                                n192 = Wait Until Next ms Multiple "Wait"(millisecond multiple=u32 250) -> ()  [unwired: 1 out]
                                n193 = Equal?(x=w259, y=w260) -> (x = y?=w261:bool)
                              }
                            }
                          }
                        }
                        frame #2 {
                          n194 = case shown="True" w268 {
                            tunnel: [_ w273] -> w267
                            tunnel: [_ w270] -> w265
                            frame False {
                            }
                            frame True {
                              n195 = local read "Detector Y Pixels"() -> (w279:i32)
                              n196 = local read "Detector X Pixels"() -> (w275:i32)
                              n197 = Multiply(x=w279, y=w275) -> (x*y=w281:i32)
                              n198 = Initialize Array "Initialize Array"(0 ("Initial values in array"), w281) -> (w283:i32[])
                              n199 = To Long Integer(number=w281) -> (32bit integer=w282:i32)
                              n200 = dll-call lib="atmcd32d.dll" fn="GetAcquiredData" label="Call Library Function Get Acquired data"(w283, w282) -> (→"Get Acquired Data":u32, w280:i32[])  [unwired: 4 in, 2 out]
                              n201 = Reshape Array(w280, w279, w275) -> (w273:i32[][])
                              n202 = call "Imageflip.vi"("2D array"=w273) -> ("transposed array"=w272:i32[][])
                              "Raw Image" <- w272
                              n203 = Transpose 2D Array(2D array=w272) -> (transposed array=w278:i32[][])
                              n204 = Array Max & Min(array=w272) -> (max value=w277:i32)  [unwired: 3 out]
                              n205 = for {
                                tunnel: w278 -> [w292] mode=indexing
                                tunnel: [w291] -> w270 mode=indexing
                                n206 = Add Array Elements(numeric array=w292) -> (sum=w291:i32)
                              }
                              "VBI" <- w270
                              n207 = Greater?(x=w277, y=64900) -> (0:w276:bool)
                              n208 = case shown="True" w276 {
                                frame False {
                                }
                                frame True {
                                n209 = local write "Camera Status:"(FALSE ("Camera Status:")) -> ()
                                n210 = property on="Camera Status:" class="Bool (strict)"("BoolText.Text"="Saturated!" ("Boolean Text.Text")) -> ()  [unwired: 2 in, 2 out]
                                n211 = Two Button Dialog(message="Camera is saturating! Reduce photon flux!", 1:"I've fixed it, and I want to continue" ("message"), 2:"Shut Down acquisition program" ("T button name (\"OK\")")) -> (T button?=w285:bool)
                                n212 = local write "Stop"(w285) -> ()
                                n213 = local write "Exit"(w285) -> ()
                                }
                              }
                            }
                          }
                          n214 = Insert Into Array(array=w266, new element=w265) -> (w264:dbl[][])  [unwired: 2 in]
                          "XUV" <- w264
                        }
                        frame #3 {
                          n215 = local read "Save image"() -> (w293:bool)
                          n216 = case shown="True" w293 {
                            tunnel: w295 -> [_ w299]
                            tunnel: w294 -> [_ w298]
                            frame False {
                            }
                            frame True {
                              n217 = Equal To 0?(x=w299) -> (x = 0?=w301:bool)
                              n218 = call "save image.vi"("Start of pump/prove run?"=w301, "Image to save"=w298, "Pump/probe run?"=TRUE) -> ("Image file path"=→"Last image saved":string)
                            }
                          }
                        }
                      }
                    }
                  }
                  frame #2 {
                    w499 = FALSE ("Start Measurement")
                    # "Free up any allocated buffers and close the camera communication channel"
                    # "Quit:"
                    # "Set the start button to false"
                    n219 = call "Cleanup.vi"("error in (no error)"=w501, "ph"=w500) -> ("error out"=w503:errorcluster, "hout"=w504:u64)  [unwired: 8 in]
                    n220 = property on="Start Measurement" class="Bool (strict)"("Value"=w499) -> ()  [unwired: 2 in, 2 out]
                    n221 = local write "Start Measurement"(w499) -> ()
                    n222 = local write "Take image"(w499) -> ()
                    n223 = local write "Run Scan"(w499) -> ()
                    n224 = call "CloseCamera.vi"("ErrorIn"=w503, "Handle in"=w504) -> ("ErrorOut"=w505:errorcluster)  [unwired: 1 in, 2 out]
                    n225 = call <vilib>:"Simple Error Handler.vi"("error in (no error)"=w505) -> ()  [unwired: 4 in, 5 out]
                    n226 = One Button Dialog(message="Measurement completed!") -> ()  [unwired: 1 in, 1 out]
                  }
                }
              }
            }
          }
        }
      }
    }
    frame #3 {
      w508 = FALSE
      n227 = flat-sequence {
        tunnel: w506 -> [w515]
        tunnel: [w515] -> w507
        tunnel: w507 -> [w517]
        frame #0 {
          n228 = local write "Camera Status:"(FALSE ("Camera Status:")) -> ()
          n229 = property on="Camera Status:" class="Bool (strict)"("BoolText.Text"="Shutting Down..." ("Boolean Text.Text")) -> ()  [unwired: 2 in, 2 out]
        }
        frame #1 {
          n230 = call "ShutDownSubVI.vi"("shutdown"=w517) -> ("Shut Down"=→"Shut Down":u32)
        }
      }
      n231 = Unbundle By Name(w509) -> ("VISA resource name"=w512:refnum<visa-resource-name>, "error"=w511:errorcluster)
      n232 = local write "Connected"(w508) -> ()
      n233 = local write "Ready"(w508) -> ()
      n234 = call <userlib>:"_Close Communications.vi"("Instrument Channel"=w512, "error in (no error)"=w511) -> ("error out"=w510:errorcluster)  [unwired: 13 in]
      n235 = call <vilib>:"General Error Handler.vi"("error in (no error)"=w510) -> ()  [unwired: 10 in, 5 out]
    }
  }
